vi "IRISS V2 Phaco v1.vi"() -> ()   [LabVIEW 2016]
uses:
  <vilib>/Analysis/Matrix/Datatypes/RealMatrix.ctl
  <vilib>/Math Plots/3D Math Plots/3D Scatter/3D Scatter XCtrl/3D Scatter.xctl
  Subsystems/Global Variables.vi
  <vilib>/Utility/file.llb/Read Delimited Spreadsheet (DBL).vi
  <vilib>/FPGAPlugInAG/PXI-7833R/niLvFpga_Open_PXI-7833R.vi
  <vilib>/Utility/error.llb/Error Cluster From Error Code.vi
  <vilib>/rvi/errors/niLvFpgaAdjustHostInterfaceError.vi
  <vilib>/Math Plots/3D Math Plots/3D Scatter/3D Scatter Datatype/Public/Plot Helper (Vector).vi
  Library/mjglib/var_OCTzHomeDir.vi
  <vilib>/FPGAPlugInAG/PXI-7833R/niLvFpga_Reset_PXI-7833R.vi
  <vilib>/FPGAPlugInAG/PXI-7833R/niLvFpga_Close_PXI-7833R.vi
  <vilib>/rvi/interface/nirviOpenFPGA/nirviOpenFPGA.xnode
  FPGA Bitfiles/PhantomControlPI_FPGATarget_QuadCtr2_E2412E44.lvbitx
  IRISS_FPGA_IO.vi
  <vilib>/rvi/interface/nirviReadWriteControl/nirviReadWriteControl.xnode
  <vilib>/Math Plots/3D Math Plots/3D Plot/3D Plot Datatype/3D Plot Datatype.lvclass
  <vilib>/rvi/interface/nirviMethod/nirviMethod.xnode
  <vilib>/rvi/interface/nirviCloseFPGA/nirviCloseFPGA.xnode
  <vilib>/Analysis/Matrix/NI_Matrix.lvlib
  Functions/EyeRobotDLL.dll
  Library/KevinLibraryAll/labview2011/kevLib2011.lvlib
  <vilib>/Math Plots/3D Math Plots/3D Scatter/3D Scatter Datatype/3D Scatter Datatype.lvclass
  NiFpgaLv.dll
panel:
  out "Trajectory Cluster":T1
  in  "OCT Z PID Gains":cluster{"Kp":dbl, "Kd":dbl, "Ki":dbl}={"Kp"=0.0003, "Kd"=0.0001, "Ki"=0.01}
  out "deltaRoll":sgl
  out "deltaXYZ":sgl[](array[numeric])
  out "Online Eye Model":T2
  in  "To Regulation":bool
  out "Eye Model Cluster":T4={"X Grid"=[], "Y Grid"=[], "Za_true Surf"=[], "Iris Center"=[], "Zp_true Surf"=[], "Pinv"=[[1.0, 0.0], [0.0, 1.0]], "za_true"=5.0, "za_work"=1.0, "zp_work"=-1.0, "zp_true"=-5.0}
  out "Update Mdl & Traj":bool=TRUE
  in  "Initialize":bool caption="To M/S"
  in  "IRISS GUI":T5(tab)
  in  "U/S Power [%]":sgl min=0 max=100 step=10
  in  "Vac Cmd [mmHg]":sgl min=0 max=600 step=50
  in  "Red Round Box":u32(colorbox)=16711690
  in  "Blue Round Box":u32(colorbox)=16860
  in  "Black Round Box":u32(colorbox)
  out "Vacuum Force [mmHg]  2":i32 caption="[mmHg]"
  in  "IV Height [mmHg]":dbl=30.0 min=0.0 max=90.0 step=10.0
  in  "Irrigation":bool
  in  "Reroute Hold [sec]":dbl=10.0 caption="Hold [sec]"
  out "Next Speed":dbl=0.8 format="%#.2gx"
  out "Current Speed":dbl=0.2 format="%#_2gx"
  out "Next Depth":dbl=40.0 format="%#_g%%"
  out "Current Depth":dbl=20.0 format="%#_6g%%"
  in  "Depth Offset":dbl min=-30.0 max=70.0 step=5.0 format="%#_g%%"
  in  "Refractive Index":dbl=1.35
  in  "PO No-Fly":dbl=5.0 step=0.1 format="%#.2g"
  out "PO Cruising":dbl=5.0 format="%#.2g"
  in  "Iris Center":dbl=5.0 step=0.1 format="%#.2g"
  in  "AN Cruising":dbl=5.0 step=0.1 format="%#.2g"
  in  "AN No-Fly":dbl=5.0 step=0.1 format="%#.2g"
  in  "Iris XY Scaling":dbl[](array[numeric])=[1.0, 1.0] caption="Iris Scaling" min=0.5 max=2.0 step=0.05
  in  "Iris XY Center":dbl[](array[numeric])=[0.0, 5.0] caption="Iris Center" min=-5.0 max=5.0 step=0.25
  out "Asgn Pt Out of Bound":bool caption="Assign Pt OOB"
  out "Emergency alarm":bool
  out "Remote sender engaged":bool
  out "State changing":bool
  out "Current Run No.":u8
  out "No. of Runs":i32=5
  out "Tip out Posit":dbl[](array[numeric]) caption="Position [mm]" format="%#.3f"
  out "Tip cmd Posit":dbl[](array[numeric]) caption="Command [mm]" format="%#.3f"
  out "State Flag Array":bool[](array[boolean])
  in  "Speed Override":u16=3
  out "Timer":i32 format="%<%M:%S>t"
  in  "Assign Point [mm]":dbl[](array[numeric])=[0.0, -7.0, -6.0]
  in  "Go to Assign Pt":bool
  out "Irrigation Engaged?":bool caption="Irrigation Engaged"
  out "Robot XYZ":refnum<class "3D Plot Datatype.lvclass">[](xcontrol)
  in  "Offset":dbl[](array[numeric])
  in  "Radial Scale":dbl=0.5
  in  "Pattern":T6(ring)=enum."Centered"
  in  "Stop-and-Go":bool
  in  "SCAN_NO":string
  in  "Gen Traj":bool
  out "Trajectory OOB":bool
  out "Current System State":T7(ring)
  in  "Current Surgical Stage":T8(ring)
  in  "Tracking Mode":u16(ring) items=["Joint Mode", "XYZ Mode"]
  in  "Stage Z [mm]":dbl=100.0 min=-120.0 max=120.0 step=0.5
  in  "Stage Y [mm]":dbl=70.0 min=-120.0 max=100.0 step=0.5
  in  "Gripper":dbl
  in  "OCT Cmd Z [mm]":dbl min=-25.0 max=14.0 step=0.5
  out "Joint Out":dbl[](array[numeric])
  out "Robot Status Array":bool[](array[boolean])
  in  "L1 [deg]":dbl=-40.0
  in  "L2 [deg]":dbl=15.0
  in  "L3 [mm]":dbl=-5.0 step=0.1
  out "Status 2":bool[](array[boolean])
  in  "L4 [deg]":dbl=-10.0 step=0.1
  in  "Home":bool
  out "OCT Z out [mm]":dbl caption="OCT Out Z [mm]" format="%#.4f"
  in  "Tool Type":i32=6
  in  "Tool Offset [mm]":dbl=-50.68
  out "Grasp out":dbl format="%#.4g"
  in  "OCTz Home Dir":bool
  in  "Remote Control Source":u16(ring) caption="Remote Source" items=["None", "Surgical Console", "Joystick", "Rigid Joystick", "Zeiss PC", "MJG C++ Teleoperation", "A-Scan", ""]
  in  "Reset Joystick":bool caption="Encoder Reset"
  out "Send Count":u64
  out "Receive Count":u64
  out "Arm ID Ind":i32
  out "Status":bool
  in  "Stage X [mm]":dbl=30.0 min=-120.0 max=120.0 step=0.5
  out "XYZ Stage out":dbl[](array[numeric])
  out "XYZ Stage cmd":dbl[](array[numeric])
  out "DH Params":cluster{"d_DH":dbl[][], "ty":dbl[][]}
  in  "Use Online Scan":bool
  in  "Process VSCAN":bool
  in  "Restart":bool
  out "Generation Error":errorcluster
  out "Model Created":bool
  in  "Eye No":i16=1 min=1 step=1
  in  "Reroute Transit Vacf":dbl=100.0
  in  "Z Rot Axis":dbl=1.0
  in  "Z Dist Thld":dbl[](array[numeric])=[3.0, 5.0] caption="Z Distance Threshould"
  in  "Vac Extremum":dbl[](array[numeric])=[68.0, 68.0] caption="Vacuum Extremum"
  in  "Max Limit [mmHg]":dbl=600.0 min=0.0 max=600.0 step=100.0
  out "Value [mmHg]":i8
  in  "Save Data":bool
  out "File Exists":bool
  out "File Path":path
  out "Elaspsed Time [s]":sgl
  in  "Data No":i16=1 min=1 step=1
  in  "Total Time":i16=90 min=1 step=1
  in  "Min PC Gap":dbl=0.1 caption="Min PC Gap [mm]" min=0.0 max=10.0 step=0.1 format="%#.3g"
  in  "Min AC Gap":dbl=0.1 caption="Min AC Gap [mm]" min=0.0 max=10.0 step=0.1 format="%#.3g"
  out "Scaling":dbl[](array[numeric])=[1.0, 1.0, 1.0] caption="S" min=0.5 max=1.5 step=0.05 format="%#_3g"
  in  "Joint Limits":dbl[][](array[numeric])=[[-68.0, -4.0], [-26.0, 52.0], [-40.0, 23.0], [-180.0, 180.0]] format="%#.3g"
  out "First Trk Pt":dbl[](array[numeric]) format="%#.3g"
  out "Error(s) Out on Program End":errorcluster
  out "L4 Waveform Graph":dbl[](graph)
  out "L3 Waveform Graph":dbl[](graph)
  out "L2 Waveform Graph":dbl[](graph)
  out "L1 Waveform Graph":dbl[](graph)
  in  "Aiming Pt":dbl[](array[numeric])=[-40.0, 11.0, 2.0, 0.0] format="%#.3g"
  in  "Engage Pt":dbl[](array[numeric])=[-40.0, 11.0, 2.0, 0.0] format="%#.3g"
  in  "Rotation":dbl[](array[numeric])=[0.0, 0.0, 0.0] caption="R [deg]" min=-15.0 max=15.0 step=0.5 format="%#_3g"
  out "Translation":dbl[](array[numeric]) caption="T [mm]" min=-3.0 max=3.0 step=0.1 format="%#_3g"
  in  "Inc Ctrl":dbl[](array[numeric])=[0.1, 0.05, 0.05] caption="Increment Control"
  in  "Depth Ctrl Array\n(% Thickness)":dbl[](array[numeric])=[40.0, 60.0, 80.0] min=10.0 max=90.0 step=5.0 format="%#_g%%"
  in  "Load Traj":bool caption="To M/S"
  in  "MS/Auto":bool
  in  "Retract":bool caption="To M/S"
  in  "Stop Accurus":bool caption="To M/S"
  in  "L3 Go Home":bool caption="To M/S"
  in  "Track":bool caption="To M/S"
  in  "Insert":bool caption="To M/S"
  in  "Program Stop":bool
  # "M/S\n \nAuto"
  # "Tool Tip Location"
  # "Tracking Planning"
  # "RCM"
  # "X\nY\nZ"
  # "X\nY\nZ"
  # "Tool"
  # "Trajectory"
  # "System Progress"
  # "Assign Point Rerouting"
  # "Trajectory Generation"
  # "X\nY\nZ"
  # "X Offset"
  # "Y Offset"
  # "Homing finished"
  # "Z Offset"
  # "M/S initialization finished"
  # "Tool Cruising Boundaries"
  # "XY-plane"
  # "Trajecoty loading finished"
  # "Aiming finished"
  # "Tool engaged"
  # "Z-axis"
  # "Phaco Machine"
  # "Tracking initialization finished"
  # "In Tracking"
  # "Rerouting finished"
  # "X\nY"
  # "X\nY"
  # "In regulation"
  # "Robot Control"
  # "Homing"
  # "Joint Definition"
  # "Arm"
  # "Tool"
  # "Stage"
  # "Robot Status"
  # "Joint M/S Cmd"
  # "HARDWARE_NOT_PRESENT"
  # "HARDWARE_NOT_FOUND_ALL_DRIVES"
  # "HARDWARE_SENSOR_FAULT"
  # "NOT_RUNNING"
  # "COMMUNICATION_ERROR"
  # "KINEMATICS_NO_SOLUTION"
  # "OCT Control"
  # "KINEMATICS_INSERTION_LENGTH_TOO_SMALL"
  # "COMMAND_BEYOND_JOINT_RANGE"
  # "COMMAND_TOO_LARGE"
  # "Eye Model Creation"
  # "Irrigation and Aspiration"
  # "IOP Control"
  # "Data Saving"
  # "Irrigation"
  # "Aspiration"
  # "ACh"
  # "Vitreous"
  # "Rotation & Vacuum Force Scheduling"
  # "Joint Motion & Control"
  # "Space Deform Parameters"
  # "Depth Ctrl"
  # "S"
  # "R"
  # "[deg]"
  # "T"
  # "[mm]"
  # "First Track Point"
  # "AC & PC Gap"
  # "X1"
  # "[mm]"
  # "Y"
  # "[mm]"
  # "Z"
  # "[mm]"
  # "L4"
  # "[deg]"
  # "Joint Limits"
  # "Error Message"
  # "Incision"
  # "Min."
  # "Max."
  # "L1"
  # "[deg]"
  # "L1"
  # "L2"
  # "L2"
  # "[deg]"
  # "L3"
  # "[mm]"
  # "L3"
  # "L4"
  # "[deg]"
  # "L4"
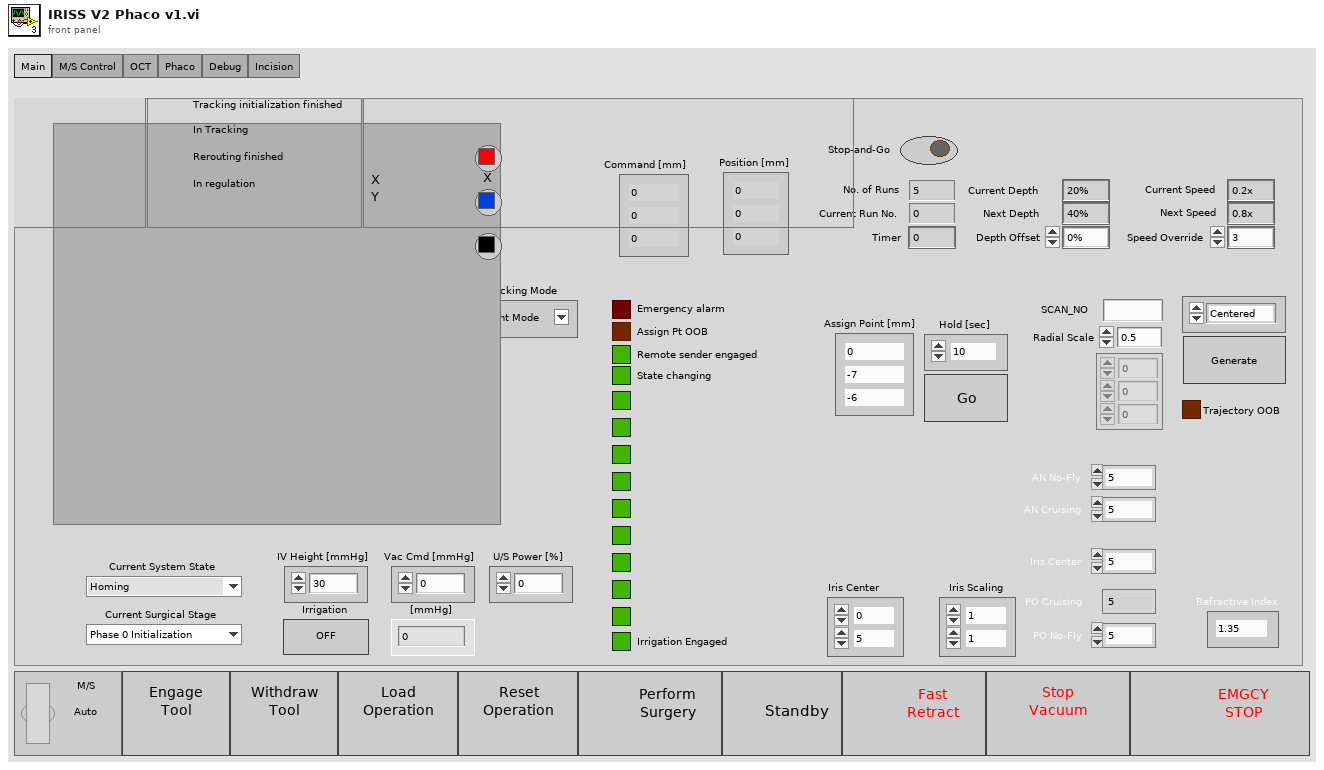
[diagram p1: front panel]
types:
  T1 = cluster{"Traj Px Array":dbl[], "Traj Py Array":dbl[], "Traj Pz Array":dbl[], "Speed Array":dbl[], "Depth Array":dbl[], "Traj Joint1 Array":dbl[], "Traj Joint2 Array":dbl[], "Traj Joint3 Array":dbl[], "Traj Joint4 Array":dbl[], "Traj Joint5 Array":dbl[]}
  T2 = cluster{"za_true":dbl, "za_work":dbl, "zi":dbl, "zp_work":dbl, "zp_true":dbl, "Iris XY Center":dbl[], "Iris XY Scaling":dbl[]}
  T3 = typedef "NI_Matrix.lvlib/RealMatrix.ctl" = dbl[][]
  T4 = cluster{"X Grid":dbl[], "Y Grid":dbl[], "Za_true Surf":dbl[][], "Iris Center":dbl[], "Zp_true Surf":dbl[][], "Pinv":T3, "za_true":dbl, "za_work":dbl, "zp_work":dbl, "zp_true":dbl}
  T5 = enum32{"Main", "M/S Control", "OCT", "Phaco", "Debug", "Incision"}
  T6 = enum16{"Entry Site", "Centered", "Insertion", "Extraction", "Reverse Entry Site", "Reverse Centered"}
  T7 = enum16{"Homing", "M/S Initialization", "M/S Operation", "Aiming", "Engaging", "Trajectory Loading", "Tracking Initialization", "Tracking", "Rerouting", "Regulation"}
  T8 = enum16{"Phase 0 Initialization", "Phase 1 Phaco", "Phase 2 Lens Removal", "Phase 3 IOL Injection"}
  T9 = enum8{"Enabled", "Disabled", "Disabled and Grayed Out"}
  T10 = cluster{"za_true_0":dbl, "za_work_0":dbl, "zp_work_0":dbl, "zp_true_0":dbl, "IrisCenter_0":dbl[]}
  T11 = cluster{"X Grid":dbl[], "Y Grid":dbl[], "Za_true Surf":dbl[][], "Iris Center":dbl[], "Zp_true Surf":dbl[][], "Real Matrix":T3, "za_true":dbl, "za_work":dbl, "zp_work":dbl, "zp_true":dbl}
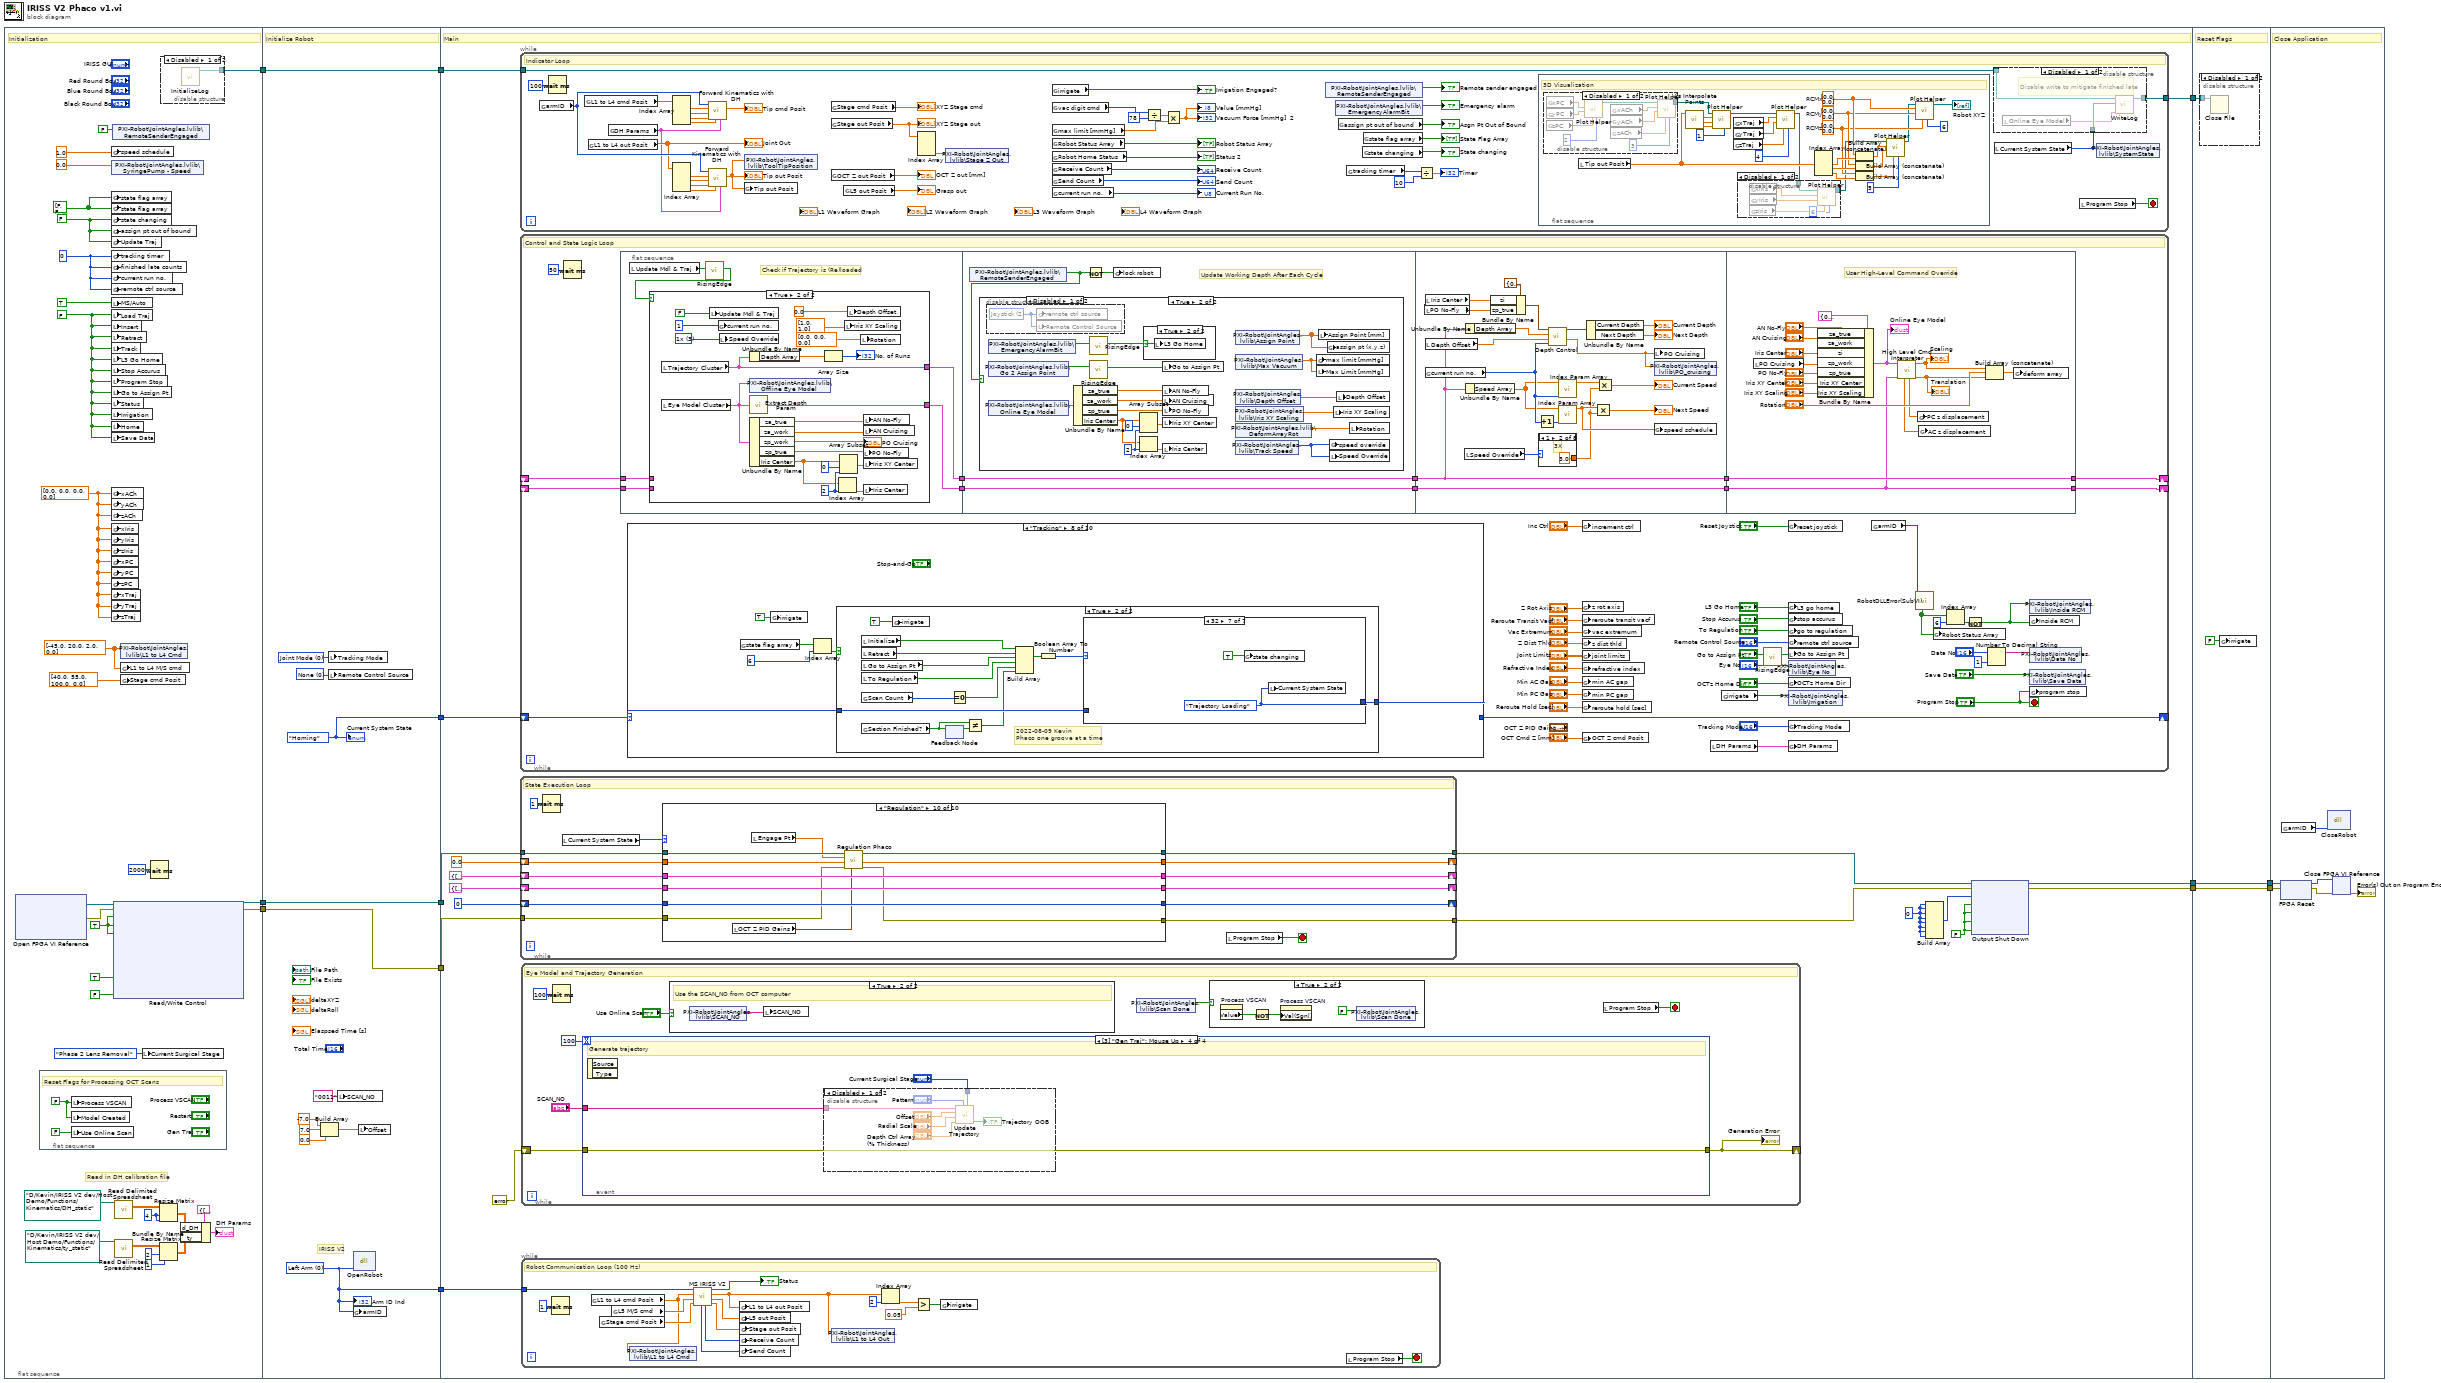
[diagram p0: block diagram]
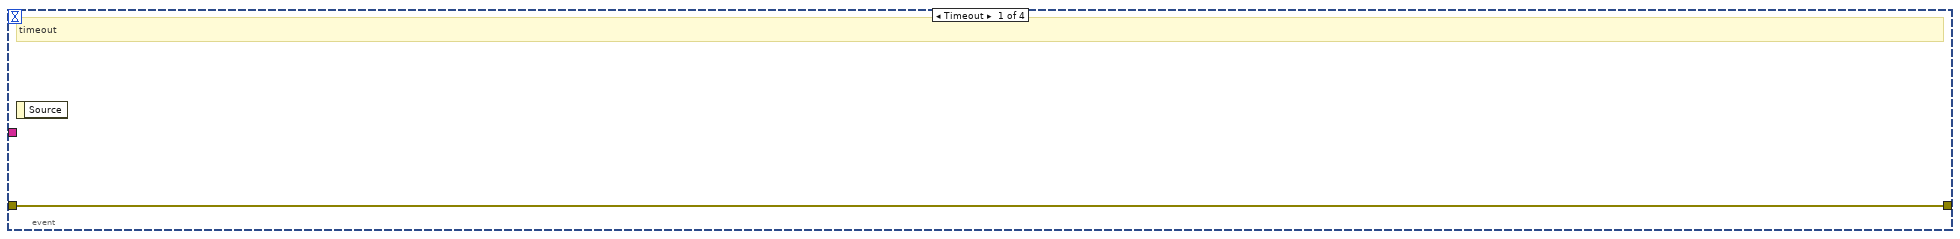
[diagram p5: hidden frame]
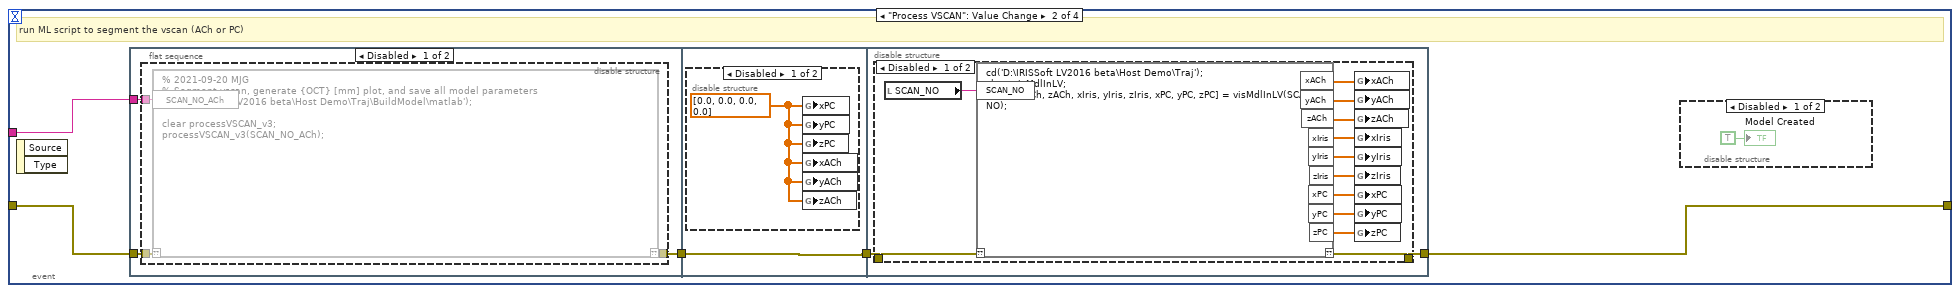
[diagram p6: hidden frame]
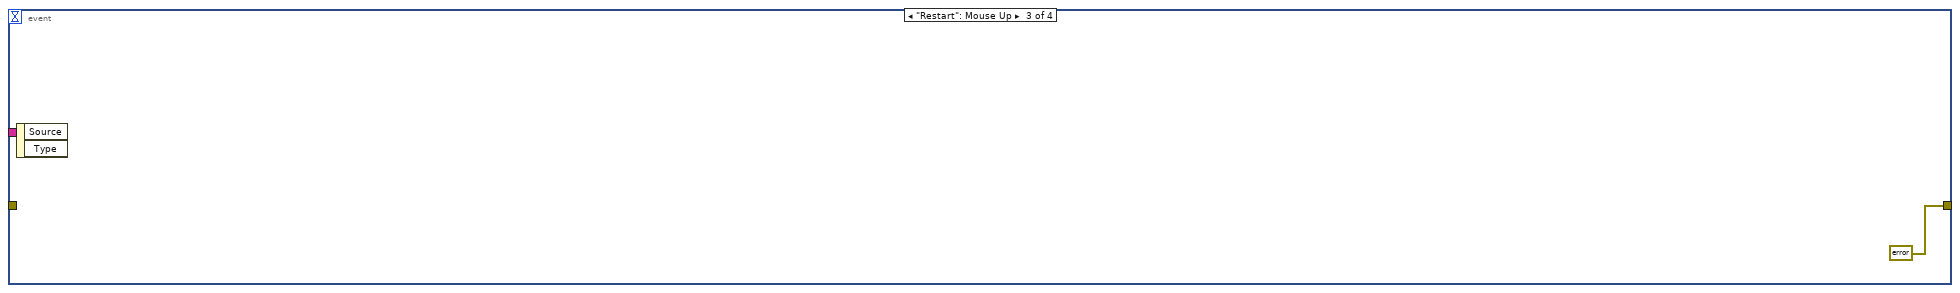
[diagram p11: hidden frame]
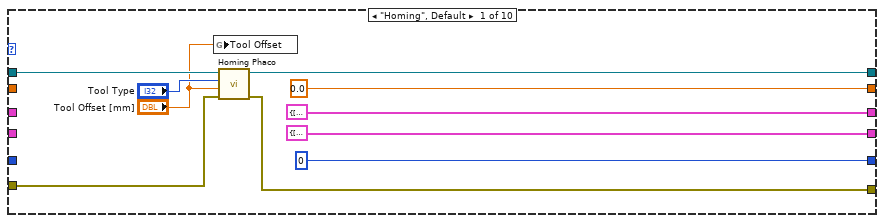
[diagram p13: hidden frame]
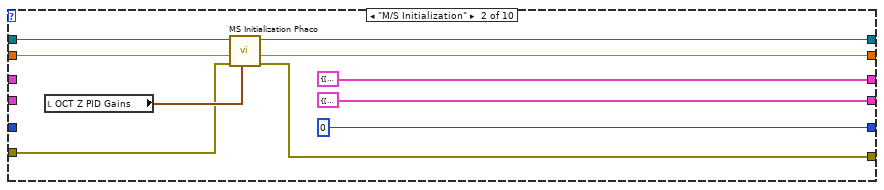
[diagram p14: hidden frame]
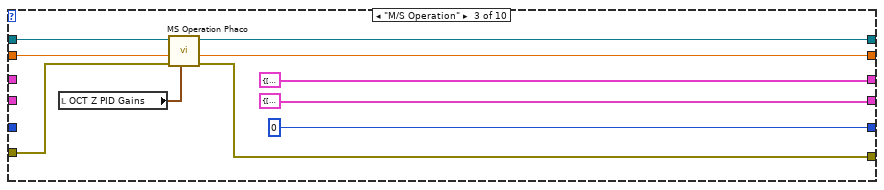
[diagram p15: hidden frame]
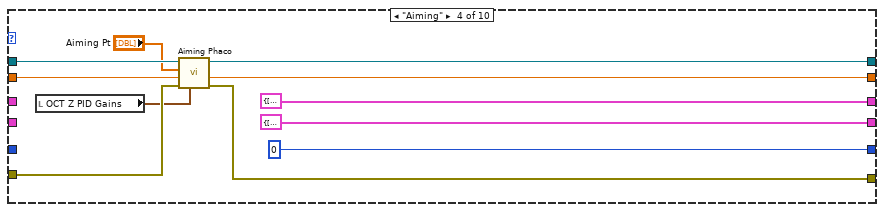
[diagram p16: hidden frame]
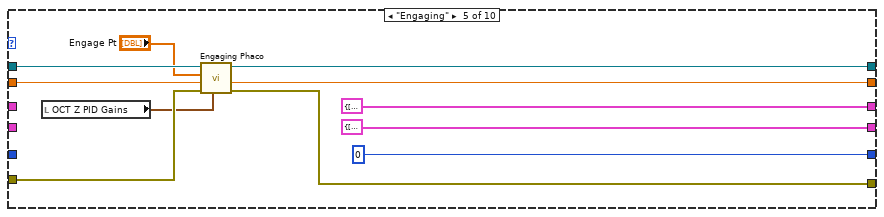
[diagram p17: hidden frame]
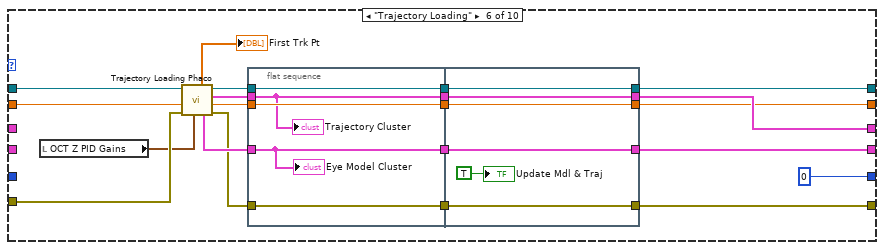
[diagram p18: hidden frame]
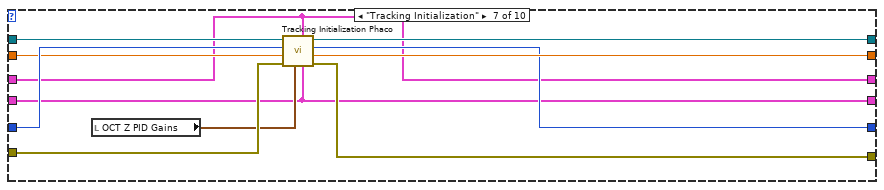
[diagram p19: hidden frame]
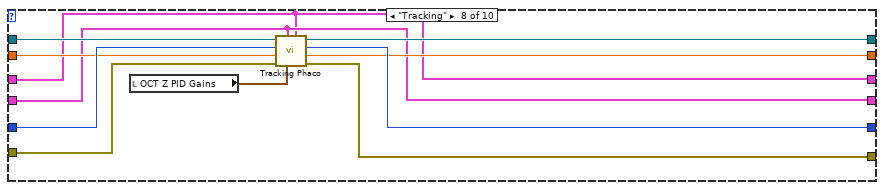
[diagram p20: hidden frame]
diagram:
  n1 = flat-sequence {
    tunnel: [w44] -> w5
    tunnel: [w36] -> w3
    tunnel: [w35] -> w2
    tunnel: [w58] -> w8
    tunnel: [w59] -> w7
    tunnel: [w57] -> w6
    tunnel: w5 -> [w60]
    tunnel: [w60] -> w4
    tunnel: w3 -> [w59]
    tunnel: w2 -> [w58]
    tunnel: [w50] -> w1
    tunnel: w8 -> [w75]
    tunnel: w7 -> [w72]
    tunnel: w6 -> [w78]
    tunnel: [w73] -> w13
    tunnel: [w74] -> w12
    tunnel: w4 -> [w77]
    tunnel: [w76] -> w11
    tunnel: w1 -> [w63]
    tunnel: w13 -> [w818]
    tunnel: w12 -> [w819]
    tunnel: w11 -> [w820]
    tunnel: [w819] -> w10
    tunnel: [w818] -> w9
    tunnel: w10 -> [w827]
    tunnel: w9 -> [w826]
    frame #0 {
      w22 = 4 ("number of rows")
      w37 = TRUE ("Conn0/DIO13 Button 2")
      w33 = dbl[] [0.0, 0.0, 0.0, 0.0] ("First Trk Pt 2")
      w28 = dbl[] [-45.0, 20.0, 2.0, 0.0] ("First Trk Pt 2")
      w32 = 0 ("finished late counts")
      w43 = bool[] [FALSE, FALSE, FALSE, FALSE, FALSE, FALSE, FALSE, FALSE, FALSE] ("state flag array")
      w41 = FALSE ("state changing")
      w34 = FALSE ("program stop")
      # "Read in DH calibration file"
      # "Initialization"
      n2 = xnode "Open FPGA VI Reference"() -> ("FPGA VI Reference Out"=w31:refnum<k20>, "error out"=w30:errorcluster)  [unwired: 2 in]
      n3 = flat-sequence {
        frame #0 {
          w46 = FALSE ("ACh Processed")
          # "Reset Flags for Processing OCT Scans"
          n4 = local write "Process VSCAN"(w46) -> ()
          n5 = local write "Model Created"(w46) -> ()
          n6 = local write "Use Online Scan"(FALSE ("Use Online Scan")) -> ()
        }
      }
      n7 = global write "Global Variables.vi" "speed schedule"(1.0 ("speed schedule")) -> ()
      n8 = shared-variable "PXI-Robot\\JointAngles.lvlib\\SyringePump - Speed"(0.0 ("SyringePump - Speed")) -> ()  [unwired: 1 in, 1 out]
      n9 = global write "Global Variables.vi" "state flag array"(w43) -> ()
      n10 = global write "Global Variables.vi" "state flag array"(w43) -> ()
      n11 = global write "Global Variables.vi" "state changing"(w41) -> ()
      n12 = global write "Global Variables.vi" "assign pt out of bound"(w41) -> ()
      n13 = global write "Global Variables.vi" "Update Traj"(w41) -> ()
      n14 = global write "Global Variables.vi" "tracking timer"(w32) -> ()
      n15 = global write "Global Variables.vi" "finished late counts"(w32) -> ()
      n16 = global write "Global Variables.vi" "current run no."(w32) -> ()
      n17 = global write "Global Variables.vi" "remote ctrl source"(w32) -> ()
      n18 = local write "MS/Auto"(TRUE ("MS/Auto")) -> ()
      n19 = local write "Load Traj"(w34) -> ()
      n20 = local write "Insert"(w34) -> ()
      n21 = local write "Retract"(w34) -> ()
      n22 = local write "Track"(w34) -> ()
      n23 = local write "L3 Go Home"(w34) -> ()
      n24 = local write "Stop Accurus"(w34) -> ()
      n25 = local write "Program Stop"(w34) -> ()
      n26 = local write "Go to Assign Pt"(w34) -> ()
      n27 = local write "Status"(w34) -> ()
      n28 = local write "Irrigation"(w34) -> ()
      n29 = local write "Home"(w34) -> ()
      n30 = local write "Save Data"(w34) -> ()
      n31 = global write "Global Variables.vi" "xACh"(w33) -> ()
      n32 = global write "Global Variables.vi" "yACh"(w33) -> ()
      n33 = global write "Global Variables.vi" "zACh"(w33) -> ()
      n34 = global write "Global Variables.vi" "xIris"(w33) -> ()
      n35 = global write "Global Variables.vi" "yIris"(w33) -> ()
      n36 = global write "Global Variables.vi" "zIris"(w33) -> ()
      n37 = global write "Global Variables.vi" "xPC"(w33) -> ()
      n38 = global write "Global Variables.vi" "yPC"(w33) -> ()
      n39 = global write "Global Variables.vi" "zPC"(w33) -> ()
      n40 = global write "Global Variables.vi" "xTraj"(w33) -> ()
      n41 = global write "Global Variables.vi" "yTraj"(w33) -> ()
      n42 = global write "Global Variables.vi" "zTraj"(w33) -> ()
      n43 = shared-variable "PXI-Robot\\JointAngles.lvlib\\RemoteSenderEngaged"(FALSE ("RemoteSenderEngaged")) -> ()  [unwired: 1 in, 1 out]
      n44 = xnode "Read/Write Control"("FPGA VI Reference In"=w31, "error in"=w30, "Conn0/DIO12 Button 1"=w37, "Conn0/DIO13 Button 2"=w37, "Conn0/DIO15 Button 4"=w37, "Reset 14"=TRUE, "Hydration On/Off (Connector2/DIO28)"=FALSE) -> ("FPGA VI Reference Out"=w36:refnum<k20>, "error out"=w35:errorcluster)  [unwired: 3 in, 2 out]
      n45 = call-poly <vilib>:"Read Delimited Spreadsheet.vi"("file path (dialog if empty)"=path "D:/Kevin/IRISS V2 dev/Host Demo/Functions/Kinematics/DH_static" ("file path (use dialog)")) -> ("all rows"=w23:dbl[][])  [unwired: 9 in, 5 out]
      n46 = call-poly <vilib>:"Read Delimited Spreadsheet.vi"("file path (dialog if empty)"=path "D:/Kevin/IRISS V2 dev/Host Demo/Functions/Kinematics/ty_static" ("file path (use dialog)")) -> ("all rows"=w21:dbl[][])  [unwired: 9 in, 5 out]
      n47 = shared-variable "PXI-Robot\\JointAngles.lvlib\\L1 to L4 Cmd"(w28) -> ()  [unwired: 1 in, 1 out]
      n48 = global write "Global Variables.vi" "L1 to L4 M/S cmd"(w28) -> ()
      n49 = global write "Global Variables.vi" "Stage cmd Posit"(dbl[] [40.0, 55.0, 100.0, 0.0] ("First Trk Pt 2")) -> ()
      n50 = local write "Current Surgical Stage"(T8."Phase 2 Lens Removal" ("Current Surgical Stage")) -> ()
      n51 = Wait (ms)(milliseconds to wait=u32 2000) -> ()  [unwired: 1 out]
      n52 = Resize Matrix(1:w22, 2:w22, 4:w23) -> (0:w17:dbl[][])
      n53 = Resize Matrix(1:1 ("number of columns"), 2:2 ("number of rows"), 4:w21) -> (0:w16:dbl[][])
      n54 = disable-structure shown="Disabled" {
        disable-tunnel: [w48 _] -> w44
        frame Disabled {
          n55 = call "InitializeLog.vi"() -> ("Byte Stream File out"=w48:refnum<file>)  [unwired: 11 in]
        }
        frame Enabled {
        }
      }
      n56 = Bundle By Name(cluster=cluster{"d_DH":dbl[][], "ty":dbl[][]} {"d_DH"=[[0.0, -0.04858099004841317, 1.1971672750675049, 0.0], [0.0, -1.576475511297109, 0.0, 0.0], [-0.3552491783526254, 0.0, -1.1064589410656984, 0.2058446720735121], [-1.0573457532495087, 1.0278049025155533, 0.011917110633363169, -0.004023577880993236]], "ty"=[[0.04320445582455471], [0.011728642746432275]]} ("input cluster"), "d_DH"=w17, "ty"=w16) -> (→"DH Params":cluster{"d_DH":dbl[][], "ty":dbl[][]})
    }
    frame #1 {
      w49 = u16 0 items=["Joint Mode", "XYZ Mode"] ("Tracking Mode")
      w56 = u16 0 items=["None", "Surgical Console", "Joystick", "MJG Teleoperation", "MJG C++ Teleoperation"] ("Remote Control Source 2")
      w57 = T7."Homing" ("Current State")
      w50 = 0 items=["Left Arm", "Right Arm"] ("Left or Right Arm")
      # "IRISS V2"
      # "Initialize Robot"
      n57 = Build Array(-7.0 ("element"), 7.0 ("element"), 0.0 ("element")) -> (w55:dbl[])
      n58 = local write "Tracking Mode"(w49) -> ()
      n59 = local write "Remote Control Source"(w56) -> ()
      n60 = local write "SCAN_NO"("0011" ("SCAN_NO")) -> ()
      n61 = dll-call lib="D:/Kevin/IRISS V2 dev/Host Demo/Functions/EyeRobotDLL.dll" fn="OpenRobot" label="Open"("id"=w50) -> ()  [unwired: 5 in, 2 out]
      n62 = global write "Global Variables.vi" "armID"(w50) -> ()
      n63 = local write "Offset"(w55) -> ()
      "Arm ID Ind" <- w50
      "Current System State" <- w57
    }
    frame #2 {
      w66 = FALSE
      w64 = i16 0 ("element")
      # "Main"
      n64 = while {
        shift-right: [w415] -> _
        shift-left: w78 -> [w416]
        shift-right: [w412] -> _
        shift-left: _ -> [w410]
        shift-right: [w411] -> _
        shift-left: _ -> [w409]
        stop <- "Program Stop" stop-if-true
        # "Control and State Logic Loop"
        n65 = Wait (ms)(milliseconds to wait=u32 50) -> ()  [unwired: 1 out]
        n66 = flat-sequence {
          tunnel: [w429] -> w401
          tunnel: [w428] -> w400
          tunnel: w410 -> [w427]
          tunnel: w409 -> [w426]
          tunnel: w401 -> [w457]
          tunnel: w400 -> [w456]
          tunnel: [w457] -> w399
          tunnel: [w456] -> w398
          tunnel: w399 -> [w485]
          tunnel: [w485] -> w397
          tunnel: w398 -> [w502]
          tunnel: [w502] -> w396
          tunnel: w397 -> [w525]
          tunnel: w396 -> [w515]
          tunnel: [w515] -> w411
          tunnel: [w525] -> w412
          frame #0 {
            # "Check if Trajectory is (Re)loaded"
            n67 = local read "Update Mdl & Traj"() -> (w431:bool)
            n68 = call "RisingEdge.vi"("Signal In"=w431) -> ("Rising Edge"=w430:bool)  [unwired: 10 in]
            n69 = case shown="True" w430 {
              tunnel: [w432 w453] -> w428
              tunnel: [w433 w442] -> w429
              tunnel: w427 -> [w433 _]
              tunnel: w426 -> [w432 _]
              frame False {
                # "Use Nominal Model & Trajectory"
              }
              frame True {
                w435 = u16 3 items=["4x", "3x", "2x", "1x", "0.5x", "0.2x", "0.1x", "PAUSE"] ("Speed Override")
                w447 = 2 ("index")
                # "Update Trajectory and Model after \"Trajectory Loading\""
                n70 = local read "Trajectory Cluster"() -> (w442:T1)
                n71 = local read "Eye Model Cluster"() -> (w440:T4)
                n72 = local write "Update Mdl & Traj"(FALSE ("Update Model")) -> ()
                n73 = global write "Global Variables.vi" "current run no."(u8 1 ("current run no.")) -> ()
                n74 = local write "Speed Override"(w435) -> ()
                n75 = Unbundle By Name(w442) -> ("Depth Array"=w444:dbl[])
                n76 = shared-variable "PXI-Robot\\JointAngles.lvlib\\Offline Eye Model"(w440) -> ()  [unwired: 1 in, 1 out]
                n77 = call "Extract Depth Param.vi"("Eye Model Cluster"=w440) -> ("Nominal Model param"=w453:T10)
                n78 = Unbundle By Name(w440) -> ("za_true"=w452:dbl, "za_work"=w451:dbl, "zp_work"=→"PO Cruising":dbl, "zp_true"=w449:dbl, "Iris Center"=w446:dbl[])
                n79 = Array Size(array=w444) -> (size(s)=→"No. of Runs":i32)
                n80 = Index Array(array=w446, index=w447) -> (element=w450:dbl)
                n81 = Array Subset(array=w446, index=0, length=w447) -> (w445:dbl[])
                n82 = local write "Iris XY Scaling"(dbl[] [1.0, 1.0]) -> ()
                n83 = local write "Depth Offset"(0.0 ("Depth Offset")) -> ()
                n84 = local write "Rotation"(dbl[] [0.0, 0.0, 0.0]) -> ()
                n85 = local write "PO No-Fly"(w449) -> ()
                n86 = local write "AN No-Fly"(w452) -> ()
                n87 = local write "AN Cruising"(w451) -> ()
                n88 = local write "Iris XY Center"(w445) -> ()
                n89 = local write "Iris Center"(w450) -> ()
              }
            }
          }
          frame #1 {
            # "Update Working Depth After Each Cycle"
            n90 = shared-variable "PXI-Robot\\JointAngles.lvlib\\RemoteSenderEngaged"() -> (w454:bool)  [unwired: 1 in, 1 out]
            n91 = case shown="True" w454 {
              frame False {
                n92 = global write "Global Variables.vi" "assign pt (x,y,z)"("Assign Point [mm]") -> ()
                n93 = global write "Global Variables.vi" "max limit [mmHg]"("Max Limit [mmHg]") -> ()
                n94 = global write "Global Variables.vi" "speed override"("Speed Override") -> ()
              }
              frame True {
                w465 = 2 ("index")
                n95 = disable-structure shown="Disabled" {
                  frame Disabled {
                    w480 = u16 2 items=["None", "Surgical Console", "Joystick", "MJG Teleoperation", "MJG C++ Teleoperation"] ("Remote Control Source 2")
                    n96 = global write "Global Variables.vi" "remote ctrl source"(w480) -> ()
                    n97 = local write "Remote Control Source"(w480) -> ()
                  }
                  frame Enabled {
                  }
                }
                n98 = shared-variable "PXI-Robot\\JointAngles.lvlib\\EmergencyAlarmBit"() -> (w477:bool)  [unwired: 1 in, 1 out]
                n99 = shared-variable "PXI-Robot\\JointAngles.lvlib\\Go 2 Assign Point"() -> (w474:bool)  [unwired: 1 in, 1 out]
                n100 = shared-variable "PXI-Robot\\JointAngles.lvlib\\Online Eye Model"() -> (w470:T11)  [unwired: 1 in, 1 out]
                n101 = Unbundle By Name(w470) -> ("za_true"=w473:dbl, "za_work"=w472:dbl, "zp_true"=w471:dbl, "Iris Center"=w462:dbl[])
                n102 = call "RisingEdge.vi"("Signal In"=w477) -> ("Rising Edge"=w476:bool)  [unwired: 10 in]
                n103 = call "RisingEdge.vi"("Signal In"=w474) -> ("Rising Edge"=w475:bool)  [unwired: 10 in]
                n104 = Index Array(array=w462, index=w465) -> (element=w463:dbl)
                n105 = Array Subset(array=w462, index=0, length=w465) -> (w466:dbl[])
                n106 = case shown="True" w476 {
                  selector: w476 -> [_ w481]
                  frame False {
                  }
                  frame True {
                    n107 = local write "L3 Go Home"(w481) -> ()
                  }
                }
                n108 = local write "Go to Assign Pt"(w475) -> ()
                n109 = local write "AN No-Fly"(w473) -> ()
                n110 = local write "AN Cruising"(w472) -> ()
                n111 = local write "PO No-Fly"(w471) -> ()
                n112 = local write "Iris XY Center"(w466) -> ()
                n113 = local write "Iris Center"(w463) -> ()
                n114 = shared-variable "PXI-Robot\\JointAngles.lvlib\\Assign Point"() -> (w478:dbl[])  [unwired: 1 in, 1 out]
                n115 = shared-variable "PXI-Robot\\JointAngles.lvlib\\Max Vacuum"() -> (w461:dbl)  [unwired: 1 in, 1 out]
                n116 = shared-variable "PXI-Robot\\JointAngles.lvlib\\Depth Offset"() -> (w469:dbl)  [unwired: 1 in, 1 out]
                n117 = shared-variable "PXI-Robot\\JointAngles.lvlib\\Iris XY Scaling"() -> (w468:dbl[])  [unwired: 1 in, 1 out]
                n118 = shared-variable "PXI-Robot\\JointAngles.lvlib\\DeformArrayRot"() -> (w467:dbl[])  [unwired: 1 in, 1 out]
                n119 = shared-variable "PXI-Robot\\JointAngles.lvlib\\Track Speed"() -> (w479:u16)  [unwired: 1 in, 1 out]
                n120 = global write "Global Variables.vi" "max limit [mmHg]"(w461) -> ()
                n121 = local write "Max Limit [mmHg]"(w461) -> ()
                n122 = local write "Assign Point [mm]"(w478) -> ()
                n123 = global write "Global Variables.vi" "assign pt (x,y,z)"(w478) -> ()
                n124 = global write "Global Variables.vi" "speed override"(w479) -> ()
                n125 = local write "Speed Override"(w479) -> ()
                n126 = local write "Iris XY Scaling"(w468) -> ()
                n127 = local write "Depth Offset"(w469) -> ()
                n128 = local write "Rotation"(w467) -> ()
              }
            }
            n129 = Not(x=w454) -> (.not. x?=w455:bool)
            n130 = global write "Global Variables.vi" "lock robot"(w455) -> ()
          }
          frame #2 {
            n131 = local read "PO No-Fly"() -> (w496:dbl)
            n132 = local read "Iris Center"() -> (w497:dbl)
            n133 = local read "Depth Offset"() -> (w501:dbl)
            n134 = global read "Global Variables.vi" "current run no."() -> (w494:u8)
            n135 = local read "Speed Override"() -> (w491:u16)
            n136 = Unbundle By Name(w485) -> ("Speed Array"=w493:dbl[])
            n137 = Unbundle By Name(w485) -> ("Depth Array"=w492:dbl[])
            n138 = Bundle By Name(cluster=cluster{"zi":dbl, "zp_true":dbl} {"zi"=0.0, "zp_true"=-2.5} ("z Cluster"), "zi"=w497, "zp_true"=w496) -> (w483:cluster{"zi":dbl, "zp_true":dbl})
            n139 = Increment(x=w494) -> (x+1=w495:u8)
            n140 = case shown="1" w491 {
              tunnel: [4.0 ("y") 3.0 ("y") 2.0 ("y") 1.0 ("y") 0.5 ("y") 0.2 ("y") 0.1 ("y") 0.0 ("y")] -> w488
              frame 0 {
                # "4X"
              }
              frame 1 {
                # "3X"
              }
              frame 2 {
                # "2X"
              }
              frame 3, Default {
                # "1x"
              }
              frame 4 {
                # "0.5x"
              }
              frame 5 {
                # "0.2x"
              }
              frame 6 {
                # "0.1x"
              }
              frame 7 {
                # "Pause"
              }
            }
            n141 = call "Depth Control.vi"("Current Run No."=w494, "Depth Offset"=w501, "Depth Array"=w492, "z Cluster"=w483) -> ("zp_work"=w482:dbl, "Schedule Depth & Speed"=w500:cluster{"Next Depth":dbl, "Current Depth":dbl})  [unwired: 6 in]
            n142 = call "Index Param Array.vi"("Index"=w494, "Array Input"=w493) -> ("Index Output"=w489:dbl)  [unwired: 9 in]
            n143 = call "Index Param Array.vi"("Index"=w495, "Array Input"=w493) -> ("Index Output"=w490:dbl)  [unwired: 9 in]
            n144 = Unbundle By Name(w500) -> ("Current Depth"=→"Current Depth":dbl, "Next Depth"=→"Next Depth":dbl)
            n145 = Multiply(x=w490, y=w488) -> (x*y=→"Next Speed":dbl)
            n146 = Multiply(x=w489, y=w488) -> (x*y=→"Current Speed":dbl)
            n147 = local write "PO Cruising"(w482) -> ()
            n148 = shared-variable "PXI-Robot\\JointAngles.lvlib\\PO_cruising"(w482) -> ()  [unwired: 1 in, 1 out]
            n149 = global write "Global Variables.vi" "speed schedule"(w490) -> ()
          }
          frame #3 {
            # "User High-Level Command Override"
            n150 = local read "PO Cruising"() -> (w517:dbl)
            n151 = Bundle By Name(cluster=T2 {"za_true"=0.0, "za_work"=0.0, "zi"=0.0, "zp_work"=0.0, "zp_true"=0.0, "Iris XY Center"=[0.0, 5.0], "Iris XY Scaling"=[1.0, 1.0]} ("High Level cmd"), "za_true"="AN No-Fly", "za_work"="AN Cruising", "zi"="Iris Center", "zp_work"=w517, "zp_true"="PO No-Fly", "Iris XY Center"="Iris XY Center", "Iris XY Scaling"="Iris XY Scaling") -> (w516:T2)
            "Online Eye Model" <- w516
            n152 = call "High Level Cmd Interpreter.vi"("Nominal Model param"=w515, "High Level cmd"=w516) -> ("Translation Array"=w512:dbl[], "Scaling Array"=w511:dbl[], "PC Displacement"=w513:dbl, "AC Displacement"=w514:dbl)  [unwired: 6 in]
            "Scaling" <- w511
            "Translation" <- w512
            n153 = global write "Global Variables.vi" "PC z displacement"(w513) -> ()
            n154 = global write "Global Variables.vi" "AC z displacement"(w514) -> ()
            n155 = Build Array (concatenate)(w511, "Rotation", w512) -> (w526:dbl[])
            n156 = global write "Global Variables.vi" "deform array"(w526) -> ()
          }
        }
        n157 = case shown="\"Tracking\"" w416 {
          selector: w416 -> [w530 w537 w563 w616 w636 w662 w671 w702 w739 w767]
          tunnel: [w529 w538 w562 w615 w637 w663 w672 w703 w740 w768] -> w415
          frame "Homing", Default {
            # "State Diagram"
            n158 = global read "Global Variables.vi" "state flag array"() -> (w531:bool[])
            n159 = Index Array(array=w531, index=0) -> (element=w528:bool)
            n160 = case shown="False" w528 {
              tunnel: [w533 w535] -> w529
              tunnel: w530 -> [w533 _]
              frame False {
                # "homing in process"
              }
              frame True {
                w535 = T7."M/S Initialization" ("Current State")
                # "finish homing"
                n161 = global write "Global Variables.vi" "state changing"(TRUE ("state changing")) -> ()
                n162 = global write "Global Variables.vi" "Enforce Homing"(FALSE ("Enforce Homing")) -> ()
                n163 = local write "Current System State"(w535) -> ()
              }
            }
          }
          frame "M/S Initialization" {
            n164 = global read "Global Variables.vi" "state flag array"() -> (w540:bool[])
            n165 = Index Array(array=w540, index=1) -> (element=w539:bool)
            n166 = case shown="False" w539 {
              tunnel: [w551 w553] -> w538
              tunnel: w537 -> [w551 _]
              frame False {
                n167 = global read "Global Variables.vi" "Stage cmd Posit"() -> (w545:dbl[])
                n168 = property on="MS/Auto" class="Bool (strict)"("DisabledEnum"=T9."Disabled and Grayed Out" ("Disabled")) -> ()  [unwired: 2 in, 2 out]
                n169 = Index Array(array=w545) -> (element #1=w543:dbl, element #2=w544:dbl, element #3=w542:dbl)  [unwired: 3 in]
                n170 = global read "Global Variables.vi" "L1 to L4 M/S cmd"() -> (w550:dbl[])
                n171 = local write "Stage X [mm]"(w543) -> ()
                n172 = local write "Stage Y [mm]"(w544) -> ()
                n173 = local write "Stage Z [mm]"(w542) -> ()
                n174 = Index Array(array=w550) -> (element #1=w549:dbl, element #2=w548:dbl, element #3=w547:dbl, element #4=w546:dbl)  [unwired: 4 in]
                n175 = local write "L1 [deg]"(w549) -> ()
                n176 = local write "L2 [deg]"(w548) -> ()
                n177 = local write "L3 [mm]"(w547) -> ()
                n178 = local write "L4 [deg]"(w546) -> ()
              }
              frame True {
                w553 = T7."M/S Operation" ("Current State")
                n179 = global write "Global Variables.vi" "state changing"(TRUE ("state changing")) -> ()
                n180 = property on="MS/Auto" class="Bool (strict)"("DisabledEnum"=T9."Enabled" ("Disabled")) -> ()  [unwired: 2 in, 2 out]
                n181 = local write "Current System State"(w553) -> ()
              }
            }
          }
          frame "M/S Operation" {
            n182 = local read "MS/Auto"() -> (w561:bool)
            n183 = local read "Load Traj"() -> (w559:bool)
            n184 = Not(x=w561) -> (.not. x?=w560:bool)
            n185 = Build Array(w560, w559, "Home") -> (w558:bool[])
            n186 = Boolean Array To Number(Boolean array=w558) -> (number=w557:u32)
            n187 = case shown="0, Default" w557 {
              tunnel: w563 -> [w566 _ w606 _]
              tunnel: [w566 w602 w607 w614] -> w562
              frame 0, Default {
                n188 = global read "Global Variables.vi" "remote ctrl source"() -> (w565:u16)
                n189 = global write "Global Variables.vi" "irrigate"("Irrigation") -> ()
                n190 = case shown="0, Default" w565 {
                  frame 0, Default {
                    n191 = Build Array("L1 [deg]", "L2 [deg]", "L3 [mm]", "L4 [deg]") -> (w582:dbl[])
                    n192 = Build Array("Stage X [mm]", "Stage Y [mm]", "Stage Z [mm]") -> (w587:dbl[])
                    n193 = global write "Global Variables.vi" "L1 to L4 M/S cmd"(w582) -> ()
                    n194 = global write "Global Variables.vi" "Stage cmd Posit"(w587) -> ()
                    n195 = global write "Global Variables.vi" "L5 M/S cmd"("Gripper") -> ()
                  }
                  frame 1 {
                    n196 = local read "OCT Cmd Z [mm]"() -> (w592:dbl)
                    n197 = global write "Global Variables.vi" "OCT Z cmd Posit"(w592) -> ()
                  }
                  frame 2 {
                    n198 = global read "Global Variables.vi" "Stage cmd Posit"() -> (w601:dbl[])
                    n199 = Index Array(array=w601) -> (element #1=w600:dbl, element #2=w599:dbl, element #3=w598:dbl)  [unwired: 3 in]
                    n200 = local write "Stage X [mm]"(w600) -> ()
                    n201 = local write "Stage Y [mm]"(w599) -> ()
                    n202 = local write "Stage Z [mm]"(w598) -> ()
                    n203 = global read "Global Variables.vi" "L1 to L4 cmd Posit"() -> (w593:dbl[])
                    n204 = Index Array(array=w593) -> (element #1=w596:dbl, element #2=w595:dbl, element #3=w594:dbl, element #4=w597:dbl)  [unwired: 4 in]
                    n205 = local write "L1 [deg]"(w596) -> ()
                    n206 = local write "L2 [deg]"(w595) -> ()
                    n207 = local write "L3 [mm]"(w594) -> ()
                    n208 = local write "L4 [deg]"(w597) -> ()
                  }
                  frame 3 {
                  }
                }
                n209 = disable-structure shown="Disabled" {
                  frame Disabled {
                    n210 = local read "Max Limit [mmHg]"() -> (w573:dbl)
                    n211 = In Range and Coerce(upper limit=w573, x="Vac Cmd [mmHg]", lower limit=0.0) -> (coerced(x)=w574:dbl)  [unwired: 1 out]
                    n212 = To Double Precision Float(number=w574) -> (double precision float=w575:dbl)
                    n213 = Divide(x=w575, y=w573) -> (x/y=w568:dbl)
                    n214 = Multiply(x="IV Height [mmHg]", y=1.36) -> (x*y=w579:dbl)
                    n215 = Multiply(x=w568, y=78.0) -> (x*y=w570:dbl)
                    n216 = To Long Integer(number=w579) -> (32bit integer=w580:i32)
                    n217 = To Long Integer(number="U/S Power [%]") -> (32bit integer=w576:i32)
                    n218 = To Byte Integer(number=w570) -> (8bit integer=w567:i8)
                    n219 = shared-variable "PXI-Robot\\JointAngles.lvlib\\Irrigation Height"(w580) -> ()  [unwired: 1 in, 1 out]
                    n220 = global write "Global Variables.vi" "us cmd"("U/S Power [%]") -> ()
                    n221 = shared-variable "PXI-Robot\\JointAngles.lvlib\\US Cmd"(w576) -> ()  [unwired: 1 in, 1 out]
                    n222 = shared-variable "PXI-Robot\\JointAngles.lvlib\\Vacuum Cmd"(w575) -> ()  [unwired: 1 in, 1 out]
                    n223 = global write "Global Variables.vi" "vac digit cmd"(w567) -> ()
                  }
                  frame Enabled {
                  }
                }
              }
              frame 1 {
                w602 = T7."Aiming" ("Current State")
                n224 = global write "Global Variables.vi" "state changing"(TRUE ("state changing")) -> ()
                n225 = local write "Current System State"(w602) -> ()
                n226 = property on="MS/Auto" class="Bool (strict)"("DisabledEnum"=T9."Disabled and Grayed Out" ("Disabled")) -> ()  [unwired: 2 in, 2 out]
              }
              frame 2 {
                n227 = global read "Global Variables.vi" "Inside RCM"() -> (w605:bool)
                n228 = case shown="True" w605 {
                  tunnel: [w608 w609] -> w607
                  tunnel: w606 -> [w608 _]
                  frame False {
                  }
                  frame True {
                    w609 = T7."Trajectory Loading" ("Current State")
                    w610 = FALSE ("MS/Auto")
                    n229 = global write "Global Variables.vi" "state changing"(TRUE ("state changing")) -> ()
                    n230 = local write "MS/Auto"(w610) -> ()
                    n231 = local write "Load Traj"(w610) -> ()
                    n232 = local write "Current System State"(w609) -> ()
                    n233 = property on="MS/Auto" class="Bool (strict)"("DisabledEnum"=T9."Disabled and Grayed Out" ("Disabled")) -> ()  [unwired: 2 in, 2 out]
                  }
                }
              }
              frame 4 {
                w614 = T7."Homing" ("Current State")
                w613 = TRUE ("state changing")
                n234 = global write "Global Variables.vi" "state changing"(w613) -> ()
                n235 = global write "Global Variables.vi" "Enforce Homing"(w613) -> ()
                n236 = local write "Current System State"(w614) -> ()
              }
            }
          }
          frame "Aiming" {
            n237 = global read "Global Variables.vi" "state flag array"() -> (w618:bool[])
            n238 = Index Array(array=w618, index=3) -> (element=w617:bool)
            n239 = case shown="True" w617 {
              tunnel: w616 -> [w620 w624]
              tunnel: [w620 w623] -> w615
              frame False {
              }
              frame True {
                n240 = property on="MS/Auto" class="Bool (strict)"("DisabledEnum"=T9."Enabled" ("Disabled")) -> ()  [unwired: 2 in, 2 out]
                n241 = Build Array("Insert", "MS/Auto") -> (w628:bool[])
                n242 = Boolean Array To Number(Boolean array=w628) -> (number=w625:u32)
                n243 = case shown="1" w625 {
                  tunnel: w624 -> [w629 _ _]
                  tunnel: [w629 w630 w634] -> w623
                  frame 0, Default {
                  }
                  frame 1 {
                    w630 = T7."Engaging" ("Current State")
                    n244 = global write "Global Variables.vi" "state changing"(TRUE ("state changing")) -> ()
                    n245 = local write "Insert"(FALSE ("Enter")) -> ()
                    n246 = property on="MS/Auto" class="Bool (strict)"("DisabledEnum"=T9."Disabled and Grayed Out" ("Disabled")) -> ()  [unwired: 2 in, 2 out]
                    n247 = local write "Current System State"(w630) -> ()
                  }
                  frame 2 {
                    w634 = T7."M/S Initialization" ("Current State")
                    n248 = global write "Global Variables.vi" "state changing"(TRUE ("state changing")) -> ()
                    n249 = local write "Current System State"(w634) -> ()
                  }
                }
                n250 = local read "OCT Cmd Z [mm]"() -> (w621:dbl)
                n251 = global write "Global Variables.vi" "OCT Z cmd Posit"(w621) -> ()
              }
            }
          }
          frame "Engaging" {
            n252 = global read "Global Variables.vi" "state flag array"() -> (w639:bool[])
            n253 = Index Array(array=w639, index=4) -> (element=w638:bool)
            n254 = case shown="True" w638 {
              tunnel: [w642 w649] -> w637
              tunnel: w636 -> [w643 w650]
              frame False {
                n255 = local read "Retract"() -> (w641:bool)
                n256 = case shown="False" w641 {
                  tunnel: [w644 w645] -> w642
                  tunnel: w643 -> [w644 _]
                  frame False {
                  }
                  frame True {
                    w645 = T7."Aiming" ("Current State")
                    n257 = global write "Global Variables.vi" "state changing"(TRUE ("state changing")) -> ()
                    n258 = local write "Retract"(FALSE ("Retract")) -> ()
                    n259 = local write "Current System State"(w645) -> ()
                  }
                }
              }
              frame True {
                n260 = Build Array("Load Traj", "Retract") -> (w653:bool[])
                n261 = Boolean Array To Number(Boolean array=w653) -> (number=w651:u32)
                n262 = case shown="2" w651 {
                  tunnel: w650 -> [w654 _ _]
                  tunnel: [w654 w655 w658] -> w649
                  frame 0, Default {
                  }
                  frame 1 {
                    w655 = T7."Trajectory Loading" ("Current State")
                    n263 = global write "Global Variables.vi" "state changing"(TRUE ("state changing")) -> ()
                    n264 = local write "Load Traj"(FALSE ("Load Traj")) -> ()
                    n265 = local write "Current System State"(w655) -> ()
                  }
                  frame 2 {
                    w658 = T7."Aiming" ("Current State")
                    n266 = global write "Global Variables.vi" "state changing"(TRUE ("state changing")) -> ()
                    n267 = local write "Retract"(FALSE ("Load Traj")) -> ()
                    n268 = local write "Current System State"(w658) -> ()
                  }
                }
              }
            }
          }
          frame "Trajectory Loading" {
            n269 = global read "Global Variables.vi" "state flag array"() -> (w665:bool[])
            n270 = global write "Global Variables.vi" "irrigate"(TRUE ("irrigate")) -> ()
            n271 = Index Array(array=w665, index=2) -> (element=w664:bool)
            n272 = case shown="False" w664 {
              tunnel: [w667 w668] -> w663
              tunnel: w662 -> [w667 _]
              frame False {
              }
              frame True {
                w668 = T7."Tracking Initialization" ("Current State")
                n273 = global write "Global Variables.vi" "state changing"(TRUE ("state changing")) -> ()
                n274 = local write "Current System State"(w668) -> ()
              }
            }
          }
          frame "Tracking Initialization" {
            n275 = global read "Global Variables.vi" "state flag array"() -> (w674:bool[])
            n276 = Index Array(array=w674, index=5) -> (element=w673:bool)
            n277 = case shown="True" w673 {
              tunnel: [w676 w683] -> w672
              tunnel: w671 -> [w676 w682]
              frame False {
              }
              frame True {
                n278 = local read "Load Traj"() -> (w684:bool)
                n279 = local read "Retract"() -> (w678:bool)
                n280 = local read "To Regulation"() -> (w677:bool)
                n281 = Or(x="Initialize", y=w678) -> (x .or. y?=w680:bool)
                n282 = Build Array("Track", w684, w680, w677) -> (w686:bool[])
                n283 = Boolean Array To Number(Boolean array=w686) -> (number=w685:u32)
                n284 = case shown="1" w685 {
                  tunnel: [w687 w688 w691 w694 w697] -> w683
                  tunnel: w682 -> [w687 _ _ _ _]
                  frame 0, Default {
                  }
                  frame 1 {
                    w688 = T7."Tracking" ("Current State")
                    n285 = global write "Global Variables.vi" "state changing"(TRUE ("state changing")) -> ()
                    n286 = local write "Track"(FALSE ("Track")) -> ()
                    n287 = local write "Current System State"(w688) -> ()
                  }
                  frame 2 {
                    w691 = T7."Trajectory Loading" ("Current State")
                    n288 = global write "Global Variables.vi" "state changing"(TRUE ("state changing")) -> ()
                    n289 = local write "Load Traj"(FALSE ("Load Traj")) -> ()
                    n290 = local write "Current System State"(w691) -> ()
                  }
                  frame 4 {
                    w694 = T7."Engaging" ("Current State")
                    n291 = global write "Global Variables.vi" "state changing"(TRUE ("state changing")) -> ()
                    n292 = local write "Initialize"(FALSE ("Load Traj")) -> ()
                    n293 = local write "Current System State"(w694) -> ()
                  }
                  frame 8 {
                    w697 = T7."Tracking" ("Current State")
                    w698 = FALSE  # Reset
                    n294 = global write "Global Variables.vi" "state changing"(TRUE ("state changing")) -> ()
                    n295 = local write "Track"(FALSE ("Track")) -> ()
                    n296 = local write "Current System State"(w697) -> ()
                    n297 = local write "To Regulation"(w698) -> ()
                  }
                }
              }
            }
            n298 = global write "Global Variables.vi" "irrigate"(TRUE ("irrigate")) -> ()
          }
          frame "Tracking" {
            n299 = global read "Global Variables.vi" "state flag array"() -> (w705:bool[])
            n300 = global write "Global Variables.vi" "irrigate"(TRUE ("irrigate")) -> ()
            n301 = Index Array(array=w705, index=6) -> (element=w704:bool)
            n302 = case shown="True" w704 {
              tunnel: [w707 w721] -> w703
              tunnel: w702 -> [w707 w720]
              frame False {
              }
              frame True {
                # "2022-08-09 Kevin\nPhaco one groove at a time"
                n303 = local read "Initialize"() -> (w717:bool)
                n304 = local read "Retract"() -> (w714:bool)
                n305 = local read "Go to Assign Pt"() -> (w715:bool)
                n306 = local read "To Regulation"() -> (w716:bool)
                n307 = global read "Global Variables.vi" "Scan Count"() -> (w709:u64)
                n308 = global read "Global Variables.vi" "Section Finished?"() -> (w710:bool)
                n309 = global write "Global Variables.vi" "irrigate"(TRUE ("irrigate")) -> ()
                n310 = feedback #1() -> (w712:bool)  [unwired: 1 in]
                n311 = feedback-in #1(w710) -> ()
                n312 = Equal To 0?(x=w709) -> (x = 0?=w708:bool)
                n313 = Not Equal?(x=w710, y=w712) -> (x != y?=w711:bool)
                n314 = Build Array(w717, w714, w715, w716, w708, w711) -> (w719:bool[])
                n315 = Boolean Array To Number(Boolean array=w719) -> (number=w718:u32)
                n316 = case shown="32" w718 {
                  tunnel: [w722 w723 w726 w729 w732 w735 w737] -> w721
                  tunnel: w720 -> [w722 _ _ _ _ _ _]
                  frame 0, Default {
                  }
                  frame 1 {
                    w723 = T7."Engaging" ("Current State")
                    n317 = global write "Global Variables.vi" "state changing"(TRUE ("state changing")) -> ()
                    n318 = local write "Initialize"(FALSE ("Load Traj")) -> ()
                    n319 = local write "Current System State"(w723) -> ()
                  }
                  frame 2 {
                    w726 = T7."Aiming" ("Current State")
                    n320 = global write "Global Variables.vi" "state changing"(TRUE ("state changing")) -> ()
                    n321 = local write "Retract"(FALSE ("Load Traj")) -> ()
                    n322 = local write "Current System State"(w726) -> ()
                  }
                  frame 4 {
                    w729 = T7."Rerouting" ("Current State")
                    n323 = global write "Global Variables.vi" "state changing"(TRUE ("state changing")) -> ()
                    n324 = local write "Go to Assign Pt"(FALSE ("Load Traj")) -> ()
                    n325 = local write "Current System State"(w729) -> ()
                  }
                  frame 8 {
                    w732 = T7."Regulation" ("Current State")
                    n326 = global write "Global Variables.vi" "state changing"(TRUE ("state changing")) -> ()
                    n327 = local write "Current System State"(w732) -> ()
                  }
                  frame 16 {
                    w735 = T7."Regulation" ("Current State")
                    w734 = TRUE ("state changing")
                    n328 = global write "Global Variables.vi" "state changing"(w734) -> ()
                    n329 = local write "To Regulation"(w734) -> ()
                    n330 = local write "Current System State"(w735) -> ()
                  }
                  frame 32 {
                    w737 = T7."Trajectory Loading" ("Current State")
                    n331 = global write "Global Variables.vi" "state changing"(TRUE ("state changing")) -> ()
                    n332 = local write "Current System State"(w737) -> ()
                  }
                }
              }
            }
          }
          frame "Rerouting" {
            n333 = global read "Global Variables.vi" "state flag array"() -> (w742:bool[])
            n334 = Index Array(array=w742, index=7) -> (element=w741:bool)
            n335 = case shown="True" w741 {
              tunnel: [w746 w760] -> w740
              tunnel: w739 -> [w745 _]
              frame False {
                n336 = shared-variable "PXI-Robot\\JointAngles.lvlib\\EmergencyAlarmBit"() -> (w752:bool)  [unwired: 1 in, 1 out]
                n337 = local read "Initialize"() -> (w751:bool)
                n338 = local read "Retract"() -> (w744:bool)
                n339 = local read "Go to Assign Pt"() -> (w748:bool)
                n340 = Compound Arithmetic op=OR(w752, w751, w744) -> (w749:bool)
                n341 = Build Array(w749, w748) -> (w750:bool[])
                n342 = Boolean Array To Number(Boolean array=w750) -> (number=w747:u32)
                n343 = case shown="2" w747 {
                  tunnel: w745 -> [w753 _ _]
                  tunnel: [w753 w754 w757] -> w746
                  frame 0, Default {
                  }
                  frame 1 {
                    w754 = T7."Engaging" ("Current State")
                    n344 = global write "Global Variables.vi" "state changing"(TRUE ("state changing")) -> ()
                    n345 = local write "Initialize"(FALSE ("Initialize")) -> ()
                    n346 = local write "Current System State"(w754) -> ()
                  }
                  frame 2 {
                    w757 = T7."Rerouting" ("Current State")
                    n347 = global write "Global Variables.vi" "state changing"(TRUE ("state changing")) -> ()
                    n348 = local write "Go to Assign Pt"(FALSE ("Initialize")) -> ()
                    n349 = local write "Current System State"(w757) -> ()
                  }
                }
              }
              frame True {
                n350 = local read "To Regulation"() -> (w761:bool)
                n351 = case shown="False" w761 {
                  tunnel: [T7."Tracking" ("Current State") T7."Regulation" ("Current State")] -> w760
                  frame False {
                    n352 = global write "Global Variables.vi" "state changing"(TRUE ("state changing")) -> ()
                  }
                  frame True {
                    n353 = global write "Global Variables.vi" "state changing"(TRUE ("state changing")) -> ()
                  }
                }
                n354 = local write "Current System State"(w760) -> ()
              }
            }
            n355 = global write "Global Variables.vi" "irrigate"(TRUE ("irrigate")) -> ()
          }
          frame "Regulation" {
            n356 = global read "Global Variables.vi" "state flag array"() -> (w770:bool[])
            n357 = global write "Global Variables.vi" "irrigate"(TRUE ("irrigate")) -> ()
            n358 = Index Array(array=w770, index=8) -> (element=w769:bool)
            n359 = case shown="True" w769 {
              tunnel: [w779 w791] -> w768
              tunnel: w767 -> [w778 w792]
              frame False {
                n360 = local read "Initialize"() -> (w777:bool)
                n361 = local read "Retract"() -> (w776:bool)
                n362 = local read "Go to Assign Pt"() -> (w772:bool)
                n363 = Or(x=w777, y=w776) -> (x .or. y?=w775:bool)
                n364 = Build Array(w775, w772) -> (w774:bool[])
                n365 = Boolean Array To Number(Boolean array=w774) -> (number=w773:u32)
                n366 = case shown="2" w773 {
                  tunnel: w778 -> [w780 _ _]
                  tunnel: [w780 w782 w785] -> w779
                  frame 0, Default {
                  }
                  frame 1 {
                    w781 = FALSE  # Reset
                    w782 = T7."Engaging" ("Current State")
                    n367 = global write "Global Variables.vi" "state changing"(TRUE ("state changing")) -> ()
                    n368 = local write "Initialize"(FALSE ("Load Traj")) -> ()
                    n369 = local write "Current System State"(w782) -> ()
                    n370 = local write "To Regulation"(w781) -> ()
                  }
                  frame 2 {
                    w785 = T7."Rerouting" ("Current State")
                    n371 = global write "Global Variables.vi" "state changing"(TRUE ("state changing")) -> ()
                    n372 = local write "Go to Assign Pt"(FALSE ("Initialize")) -> ()
                    n373 = local write "Current System State"(w785) -> ()
                  }
                }
              }
              frame True {
                n374 = local read "Load Traj"() -> (w794:bool)
                n375 = local read "Go to Assign Pt"() -> (w795:bool)
                n376 = local read "Initialize"() -> (w790:bool)
                n377 = local read "Retract"() -> (w788:bool)
                n378 = local read "Track"() -> (w789:bool)
                n379 = Build Array(w794, w795, w790, w788, w789) -> (w796:bool[])
                n380 = Boolean Array To Number(Boolean array=w796) -> (number=w793:u32)
                n381 = case shown="8" w793 {
                  tunnel: w792 -> [w797 _ _ _ _ _]
                  tunnel: [w797 w799 w802 w806 w810 w814] -> w791
                  frame 0, Default {
                  }
                  frame 1 {
                    w798 = FALSE  # Reset
                    w799 = T7."Trajectory Loading" ("Current State")
                    n382 = global write "Global Variables.vi" "state changing"(TRUE ("state changing")) -> ()
                    n383 = local write "Load Traj"(FALSE ("Load Traj")) -> ()
                    n384 = local write "Current System State"(w799) -> ()
                    n385 = local write "To Regulation"(w798) -> ()
                  }
                  frame 2 {
                    w802 = T7."Rerouting" ("Current State")
                    n386 = global write "Global Variables.vi" "state changing"(TRUE ("state changing")) -> ()
                    n387 = local write "Go to Assign Pt"(FALSE ("Load Traj")) -> ()
                    n388 = local write "Current System State"(w802) -> ()
                  }
                  frame 4 {
                    w805 = FALSE  # Reset
                    w806 = T7."Engaging" ("Current State")
                    n389 = global write "Global Variables.vi" "state changing"(TRUE ("state changing")) -> ()
                    n390 = local write "Initialize"(FALSE ("Load Traj")) -> ()
                    n391 = local write "To Regulation"(w805) -> ()
                    n392 = local write "Current System State"(w806) -> ()
                  }
                  frame 8 {
                    w809 = FALSE  # Reset
                    w810 = T7."Aiming" ("Current State")
                    n393 = global write "Global Variables.vi" "state changing"(TRUE ("state changing")) -> ()
                    n394 = local write "Retract"(FALSE ("Load Traj")) -> ()
                    n395 = local write "To Regulation"(w809) -> ()
                    n396 = local write "Current System State"(w810) -> ()
                  }
                  frame 16 {
                    w813 = FALSE  # Reset
                    w814 = T7."Tracking" ("Current State")
                    n397 = global write "Global Variables.vi" "state changing"(TRUE ("state changing")) -> ()
                    n398 = local write "Track"(FALSE ("Load Traj")) -> ()
                    n399 = local write "Current System State"(w814) -> ()
                    n400 = local write "To Regulation"(w813) -> ()
                  }
                }
              }
            }
          }
        }
        n401 = global write "Global Variables.vi" "increment ctrl"("Inc Ctrl") -> ()
        n402 = global write "Global Variables.vi" "z rot axis"("Z Rot Axis") -> ()
        n403 = global write "Global Variables.vi" "reroute transit vacf"("Reroute Transit Vacf") -> ()
        n404 = global write "Global Variables.vi" "vac extremum"("Vac Extremum") -> ()
        n405 = global write "Global Variables.vi" "z dist thld"("Z Dist Thld") -> ()
        n406 = global write "Global Variables.vi" "joint limits"("Joint Limits") -> ()
        n407 = global write "Global Variables.vi" "refractive index"("Refractive Index") -> ()
        n408 = global write "Global Variables.vi" "min AC gap"("Min AC Gap") -> ()
        n409 = global write "Global Variables.vi" "min PC gap"("Min PC Gap") -> ()
        n410 = global write "Global Variables.vi" "reroute hold [sec]"("Reroute Hold [sec]") -> ()
        n411 = global write "Global Variables.vi" "OCT Z cmd Posit"("OCT Cmd Z [mm]") -> ()
        n412 = local read "DH Params"() -> (w380:cluster{"d_DH":dbl[][], "ty":dbl[][]})
        n413 = global read "Global Variables.vi" "irrigate"() -> (w388:bool)
        n414 = call "RisingEdge.vi"("Signal In"="Go to Assign Pt") -> ("Rising Edge"=w402:bool)  [unwired: 10 in]
        n415 = global write "Global Variables.vi" "reset joystick"("Reset Joystick") -> ()
        n416 = global write "Global Variables.vi" "L3 go home"("L3 Go Home") -> ()
        n417 = global write "Global Variables.vi" "stop accurus"("Stop Accurus") -> ()
        n418 = global write "Global Variables.vi" "go to regulation"("To Regulation") -> ()
        n419 = global write "Global Variables.vi" "remote ctrl source"("Remote Control Source") -> ()
        n420 = local write "Go to Assign Pt"(w402) -> ()
        n421 = shared-variable "PXI-Robot\\JointAngles.lvlib\\Eye No"("Eye No") -> ()  [unwired: 1 in, 1 out]
        n422 = global write "var_OCTzHomeDir.vi" "OCTz Home Dir"("OCTz Home Dir") -> ()
        n423 = shared-variable "PXI-Robot\\JointAngles.lvlib\\Irrigation"(w388) -> ()  [unwired: 1 in, 1 out]
        n424 = global write "Global Variables.vi" "Tracking Mode"("Tracking Mode") -> ()
        n425 = global write "Global Variables.vi" "DH Params"(w380) -> ()
        n426 = global read "Global Variables.vi" "armID"() -> (w394:i32)
        n427 = call "RobotDLLError(SubVI).vi"("ArmID"=w394) -> ("RobotStatusArray"=w393:bool[])  [unwired: 5 in, 9 out]
        n428 = global write "Global Variables.vi" "Robot Status Array"(w393) -> ()
        n429 = Index Array(array=w393, index=6) -> (element=w391:bool)
        n430 = Not(x=w391) -> (.not. x?=w390:bool)
        n431 = Number To Decimal String(number="Data No", width (-)=i16 1) -> (decimal integer string=w383:string)
        n432 = shared-variable "PXI-Robot\\JointAngles.lvlib\\Inside RCM"(w390) -> ()  [unwired: 1 in, 1 out]
        n433 = global write "Global Variables.vi" "Inside RCM"(w390) -> ()
        n434 = shared-variable "PXI-Robot\\JointAngles.lvlib\\Data No"(w383) -> ()  [unwired: 1 in, 1 out]
        n435 = shared-variable "PXI-Robot\\JointAngles.lvlib\\Save Data"("Save Data") -> ()  [unwired: 1 in, 1 out]
        n436 = global write "Global Variables.vi" "program stop"("Program Stop") -> ()
      }
      n437 = while {
        tunnel: w72 -> [w160]
        tunnel: w75 -> [w159]
        tunnel: [w158] -> w68
        tunnel: [w157] -> w67
        shift-right: [w155] -> _
        shift-left: 0.0 ("Prev OCT Z Posit") -> [w156]
        shift-right: [w153] -> _
        shift-left: 0 -> [w152]
        shift-right: [w151] -> _
        shift-left: T1 {"Traj Px Array"=[], "Traj Py Array"=[], "Traj Pz Array"=[], "Speed Array"=[], "Depth Array"=[], "Traj Joint1 Array"=[], "Traj Joint2 Array"=[], "Traj Joint3 Array"=[], "Traj Joint4 Array"=[], "Traj Joint5 Array"=[]} ("Trajectory Cluster 2") -> [w149]
        shift-right: [w150] -> _
        shift-left: T4 {"X Grid"=[], "Y Grid"=[], "Za_true Surf"=[], "Iris Center"=[0.0, 5.0, 0.0], "Zp_true Surf"=[], "Pinv"=[[1.0, 0.0], [0.0, 1.0]], "za_true"=0.0, "za_work"=0.0, "zp_work"=0.0, "zp_true"=0.0} ("Eye Model Cluster") -> [w148]
        stop <- w154 stop-if-true
        # "State Execution Loop"
        n438 = Wait (ms)(milliseconds to wait=u32 1) -> ()  [unwired: 1 out]
        n439 = local read "Current System State"() -> (w147:T7)
        n440 = case shown="\"Regulation\"" w147 {
          tunnel: w160 -> [w167 w178 w188 w199 w210 w223 w256 w267 w278 w286]
          tunnel: w159 -> [w163 w174 w183 w194 w205 w220 w252 w261 w272 w281]
          tunnel: [w166 w177 w187 w198 w209 w232 w255 w266 w277 w285] -> w158
          tunnel: [w162 w172 w182 w192 w203 w233 w251 w260 w271 w280] -> w157
          tunnel: w156 -> [_ w176 w185 w196 w207 w221 w253 w263 w274 w283]
          tunnel: [0.0 ("Prev OCT Z Posit") w173 w184 w195 w206 w224 w250 w262 w273 w282] -> w155
          tunnel: [0 ("Last Index") 0 ("Last Index") 0 ("Last Index") 0 ("Last Index") 0 ("Last Index") 0 w249 w264 w275 w289] -> w153
          tunnel: w152 -> [_ _ _ _ _ _ w254 w265 w276 w289]
          tunnel: [T1 {"Traj Px Array"=[], "Traj Py Array"=[], "Traj Pz Array"=[], "Speed Array"=[], "Depth Array"=[], "Traj Joint1 Array"=[], "Traj Joint2 Array"=[], "Traj Joint3 Array"=[], "Traj Joint4 Array"=[], "Traj Joint5 Array"=[]} ("Trajectory Cluster 2") T1 {"Traj Px Array"=[], "Traj Py Array"=[], "Traj Pz Array"=[], "Speed Array"=[], "Depth Array"=[], "Traj Joint1 Array"=[], "Traj Joint2 Array"=[], "Traj Joint3 Array"=[], "Traj Joint4 Array"=[], "Traj Joint5 Array"=[]} ("Trajectory Cluster 2") T1 {"Traj Px Array"=[], "Traj Py Array"=[], "Traj Pz Array"=[], "Speed Array"=[], "Depth Array"=[], "Traj Joint1 Array"=[], "Traj Joint2 Array"=[], "Traj Joint3 Array"=[], "Traj Joint4 Array"=[], "Traj Joint5 Array"=[]} ("Trajectory Cluster 2") T1 {"Traj Px Array"=[], "Traj Py Array"=[], "Traj Pz Array"=[], "Speed Array"=[], "Depth Array"=[], "Traj Joint1 Array"=[], "Traj Joint2 Array"=[], "Traj Joint3 Array"=[], "Traj Joint4 Array"=[], "Traj Joint5 Array"=[]} ("Trajectory Cluster 2") T1 {"Traj Px Array"=[], "Traj Py Array"=[], "Traj Pz Array"=[], "Speed Array"=[], "Depth Array"=[], "Traj Joint1 Array"=[], "Traj Joint2 Array"=[], "Traj Joint3 Array"=[], "Traj Joint4 Array"=[], "Traj Joint5 Array"=[]} ("Trajectory Cluster 2") w231 w248 w257 w268 w288] -> w151
          tunnel: [T4 {"X Grid"=[], "Y Grid"=[], "Za_true Surf"=[], "Iris Center"=[0.0, 5.0, 0.0], "Zp_true Surf"=[], "Pinv"=[[1.0, 0.0], [0.0, 1.0]], "za_true"=0.0, "za_work"=0.0, "zp_work"=0.0, "zp_true"=0.0} ("Eye Model Cluster") T4 {"X Grid"=[], "Y Grid"=[], "Za_true Surf"=[], "Iris Center"=[0.0, 5.0, 0.0], "Zp_true Surf"=[], "Pinv"=[[1.0, 0.0], [0.0, 1.0]], "za_true"=0.0, "za_work"=0.0, "zp_work"=0.0, "zp_true"=0.0} ("Eye Model Cluster") T4 {"X Grid"=[], "Y Grid"=[], "Za_true Surf"=[], "Iris Center"=[0.0, 5.0, 0.0], "Zp_true Surf"=[], "Pinv"=[[1.0, 0.0], [0.0, 1.0]], "za_true"=0.0, "za_work"=0.0, "zp_work"=0.0, "zp_true"=0.0} ("Eye Model Cluster") T4 {"X Grid"=[], "Y Grid"=[], "Za_true Surf"=[], "Iris Center"=[0.0, 5.0, 0.0], "Zp_true Surf"=[], "Pinv"=[[1.0, 0.0], [0.0, 1.0]], "za_true"=0.0, "za_work"=0.0, "zp_work"=0.0, "zp_true"=0.0} ("Eye Model Cluster") T4 {"X Grid"=[], "Y Grid"=[], "Za_true Surf"=[], "Iris Center"=[0.0, 5.0, 0.0], "Zp_true Surf"=[], "Pinv"=[[1.0, 0.0], [0.0, 1.0]], "za_true"=0.0, "za_work"=0.0, "zp_work"=0.0, "zp_true"=0.0} ("Eye Model Cluster") w230 w246 w258 w270 w287] -> w150
          tunnel: w149 -> [_ _ _ _ _ _ w248 w257 w268 w288]
          tunnel: w148 -> [_ _ _ _ _ _ w246 w258 w270 w287]
          frame "Homing", Default {
            n441 = global write "Global Variables.vi" "Tool Offset"("Tool Offset [mm]") -> ()
            n442 = call "Homing Phaco.vi"("error in"=w163, "Tool Offset"="Tool Offset [mm]", "ToolType"="Tool Type", "FPGA VI Reference In"=w167) -> ("error out"=w162:errorcluster, "FPGA VI Reference Out"=w166:refnum<k20>)  [unwired: 6 in]
          }
          frame "M/S Initialization" {
            n443 = local read "OCT Z PID Gains"() -> (w175:cluster{"Kp":dbl, "Kd":dbl, "Ki":dbl})
            n444 = call "MS Initialization Phaco.vi"("OCT Z PID Gains"=w175, "error in"=w174, "OCT Prev Posit"=w176, "FPGA VI Reference In"=w178) -> ("error out"=w172:errorcluster, "OCT Last Posit"=w173:dbl, "FPGA VI Reference Out"=w177:refnum<k20>)  [unwired: 5 in]
          }
          frame "M/S Operation" {
            n445 = local read "OCT Z PID Gains"() -> (w186:cluster{"Kp":dbl, "Kd":dbl, "Ki":dbl})
            n446 = call "MS Operation Phaco.vi"("OCT Z PID Gains"=w186, "error in"=w183, "OCT Prev Posit"=w185, "FPGA VI Reference In"=w188) -> ("error out"=w182:errorcluster, "OCT Last Posit"=w184:dbl, "FPGA VI Reference Out"=w187:refnum<k20>)  [unwired: 5 in]
          }
          frame "Aiming" {
            n447 = local read "OCT Z PID Gains"() -> (w193:cluster{"Kp":dbl, "Kd":dbl, "Ki":dbl})
            n448 = call "Aiming Phaco.vi"("OCT Z PID Gains"=w193, "error in"=w194, "OCT Prev Posit"=w196, "Aiming Pt"="Aiming Pt", "FPGA VI Reference In"=w199) -> ("error out"=w192:errorcluster, "OCT Last Posit"=w195:dbl, "FPGA VI Reference Out"=w198:refnum<k20>)  [unwired: 4 in]
          }
          frame "Engaging" {
            n449 = local read "OCT Z PID Gains"() -> (w204:cluster{"Kp":dbl, "Kd":dbl, "Ki":dbl})
            n450 = call "Engaging Phaco.vi"("OCT Z PID Gains"=w204, "error in"=w205, "OCT Prev Posit"=w207, "Engage Pt"="Engage Pt", "FPGA VI Reference In"=w210) -> ("error out"=w203:errorcluster, "OCT Last Posit"=w206:dbl, "FPGA VI Reference Out"=w209:refnum<k20>)  [unwired: 4 in]
          }
          frame "Trajectory Loading" {
            n451 = local read "OCT Z PID Gains"() -> (w219:cluster{"Kp":dbl, "Kd":dbl, "Ki":dbl})
            n452 = call "Trajectory Loading Phaco.vi"("OCT Z PID Gains"=w219, "error in"=w220, "OCT Prev Posit"=w221, "FPGA VI Reference In"=w223) -> ("error out"=w217:errorcluster, "OCT Last Posit"=w216:dbl, "Trajectory Cluster"=w215:T1, "FPGA VI Reference Out"=w214:refnum<k20>, "Eye Model Cluster"=w218:T4, "First Trk Pt"=→"First Trk Pt":dbl[])  [unwired: 2 in]
            n453 = flat-sequence {
              tunnel: w218 -> [w237]
              tunnel: w217 -> [w239]
              tunnel: [w239] -> w229
              tunnel: w214 -> [w238]
              tunnel: [w238] -> w228
              tunnel: [w235] -> w227
              tunnel: w215 -> [w235]
              tunnel: [w237] -> w226
              tunnel: w216 -> [w236]
              tunnel: [w236] -> w225
              tunnel: [w244] -> w233
              tunnel: w229 -> [w244]
              tunnel: w228 -> [w243]
              tunnel: [w243] -> w232
              tunnel: w227 -> [w242]
              tunnel: w226 -> [w241]
              tunnel: [w242] -> w231
              tunnel: [w241] -> w230
              tunnel: w225 -> [w240]
              tunnel: [w240] -> w224
              frame #0 {
                "Eye Model Cluster" <- w237
                "Trajectory Cluster" <- w235
              }
              frame #1 {
                "Update Mdl & Traj" <- TRUE
              }
            }
          }
          frame "Tracking Initialization" {
            n454 = local read "OCT Z PID Gains"() -> (w247:cluster{"Kp":dbl, "Kd":dbl, "Ki":dbl})
            n455 = call "Tracking Initialization Phaco.vi"("Eye Model Cluster"=w246, "Trajectory Cluster"=w248, "OCT Z PID Gains"=w247, "error in"=w252, "OCT Prev Posit"=w253, "Prev Index"=w254, "FPGA VI Reference In"=w256) -> ("error out"=w251:errorcluster, "OCT Last Posit"=w250:dbl, "Last Index"=w249:i32, "FPGA VI Reference Out"=w255:refnum<k20>)  [unwired: 1 in]
          }
          frame "Tracking" {
            n456 = local read "OCT Z PID Gains"() -> (w259:cluster{"Kp":dbl, "Kd":dbl, "Ki":dbl})
            n457 = call "Tracking Phaco.vi"("Trajectory Cluster"=w257, "OCT Z PID Gains"=w259, "Eye Model Cluster"=w258, "error in"=w261, "OCT Prev Posit"=w263, "Resume Index"=w265, "FPGA VI Reference In"=w267) -> ("error out"=w260:errorcluster, "OCT Last Posit"=w262:dbl, "Leave Index"=w264:i32, "FPGA VI Reference Out"=w266:refnum<k20>)  [unwired: 1 in]
          }
          frame "Rerouting" {
            n458 = local read "OCT Z PID Gains"() -> (w269:cluster{"Kp":dbl, "Kd":dbl, "Ki":dbl})
            n459 = call "Rerouting Phaco.vi"("Eye Model Cluster"=w270, "Trajectory Cluster"=w268, "OCT Z PID Gains"=w269, "error in"=w272, "OCT Prev Posit"=w274, "Prev Index"=w276, "FPGA VI Reference In"=w278) -> ("error out"=w271:errorcluster, "OCT Last Posit"=w273:dbl, "Last Index"=w275:i32, "FPGA VI Reference Out"=w277:refnum<k20>)  [unwired: 1 in]
          }
          frame "Regulation" {
            n460 = local read "OCT Z PID Gains"() -> (w279:cluster{"Kp":dbl, "Kd":dbl, "Ki":dbl})
            n461 = local read "Engage Pt"() -> (w284:dbl[])
            n462 = call "Regulation Phaco.vi"("OCT Z PID Gains"=w279, "error in"=w281, "OCT Prev Posit"=w283, "Engage Pt"=w284, "FPGA VI Reference In"=w286) -> ("error out"=w280:errorcluster, "OCT Last Posit"=w282:dbl, "FPGA VI Reference Out"=w285:refnum<k20>)  [unwired: 4 in]
          }
        }
        n463 = local read "Program Stop"() -> (w154:bool)
      }
      n464 = while {
        tunnel: w77 -> [w322]
        tunnel: [w321] -> w76
        stop <- w331 stop-if-true
        # "Indicator Loop"
        n465 = global read "Global Variables.vi" "armID"() -> (w297:i32)
        n466 = Wait (ms)(milliseconds to wait=u32 100) -> ()  [unwired: 1 out]
        n467 = global read "Global Variables.vi" "L1 to L4 cmd Posit"() -> (w303:dbl[])
        n468 = global read "Global Variables.vi" "L1 to L4 out Posit"() -> (w296:dbl[])
        "Joint Out" <- w296
        n469 = global read "Global Variables.vi" "DH Params"() -> (w290:cluster{"d_DH":dbl[][], "ty":dbl[][]})
        n470 = Index Array(array=w303) -> (element #1=w302:dbl, element #2=w301:dbl, element #3=w300:dbl, element #4=w298:dbl)  [unwired: 4 in]
        n471 = Index Array(array=w296) -> (element #1=w295:dbl, element #2=w294:dbl, element #3=w293:dbl, element #4=w292:dbl)  [unwired: 4 in]
        n472 = call "Forward Kinematics with DH.vi"("DH Params"=w290, "j4"=w298, "j3"=w300, "j2"=w301, "j1"=w302, "armID"=w297) -> ("XYZ With DH Calibration"=→"Tip cmd Posit":dbl[])  [unwired: 5 in]
        n473 = call "Forward Kinematics with DH.vi"("DH Params"=w290, "j4"=w292, "j3"=w293, "j2"=w294, "j1"=w295, "armID"=w297) -> ("XYZ With DH Calibration"=w291:dbl[])  [unwired: 5 in]
        "Tip out Posit" <- w291
        n474 = shared-variable "PXI-Robot\\JointAngles.lvlib\\ToolTipPosition"(w291) -> ()  [unwired: 1 in, 1 out]
        n475 = global write "Global Variables.vi" "Tip out Posit"(w291) -> ()
        n476 = global read "Global Variables.vi" "Stage cmd Posit"() -> (→"XYZ Stage cmd":dbl[])
        n477 = global read "Global Variables.vi" "Stage out Posit"() -> (w306:dbl[])
        "XYZ Stage out" <- w306
        n478 = global read "Global Variables.vi" "OCT Z out Posit"() -> (→"OCT Z out [mm]":dbl)
        n479 = global read "Global Variables.vi" "L5 out Posit"() -> (→"Grasp out":dbl)
        n480 = Index Array(array=w306) -> (element #3=w307:dbl)  [unwired: 3 in, 2 out]
        n481 = shared-variable "PXI-Robot\\JointAngles.lvlib\\Stage Z Out"(w307) -> ()  [unwired: 1 in, 1 out]
        n482 = global read "Global Variables.vi" "irrigate"() -> (→"Irrigation Engaged?":bool)
        n483 = global read "Global Variables.vi" "vac digit cmd"() -> (w312:i8)
        n484 = global read "Global Variables.vi" "max limit [mmHg]"() -> (w309:dbl)
        n485 = global read "Global Variables.vi" "Robot Status Array"() -> (→"Robot Status Array":bool[])
        n486 = global read "Global Variables.vi" "Robot Home Status"() -> (→"Status 2":bool[])
        n487 = global read "Global Variables.vi" "Receive Count"() -> (→"Receive Count":u64)
        n488 = global read "Global Variables.vi" "Send Count"() -> (→"Send Count":u64)
        n489 = global read "Global Variables.vi" "current run no."() -> (→"Current Run No.":u8)
        n490 = Divide(x=w312, y=i8 78) -> (x/y=w310:dbl)
        n491 = Multiply(x=w310, y=w309) -> (x*y=→"Value [mmHg]" →"Vacuum Force [mmHg]  2":dbl)
        n492 = shared-variable "PXI-Robot\\JointAngles.lvlib\\RemoteSenderEngaged"() -> (→"Remote sender engaged":bool)  [unwired: 1 in, 1 out]
        n493 = shared-variable "PXI-Robot\\JointAngles.lvlib\\EmergencyAlarmBit"() -> (→"Emergency alarm":bool)  [unwired: 1 in, 1 out]
        n494 = global read "Global Variables.vi" "assign pt out of bound"() -> (→"Asgn Pt Out of Bound":bool)
        n495 = global read "Global Variables.vi" "tracking timer"() -> (w324:i32)
        n496 = global read "Global Variables.vi" "state changing"() -> (→"State changing":bool)
        n497 = global read "Global Variables.vi" "state flag array"() -> (→"State Flag Array":bool[])
        n498 = Divide(x=w324, y=10) -> (x/y=→"Timer":dbl)
        n499 = flat-sequence {
          frame #0 {
            w353 = sgl[] [0.0, 0.0]  # RCMy
            w352 = sgl[] [0.0, 0.0]  # RCMz
            w354 = sgl[] [0.0, 0.0]  # RCMx
            # "3D Visualization"
            n500 = disable-structure shown="Disabled" {
              disable-tunnel: [w363 _] -> w342
              frame Disabled {
                n501 = global read "Global Variables.vi" "xPC"() -> (w361:dbl[])
                n502 = global read "Global Variables.vi" "yPC"() -> (w360:dbl[])
                n503 = global read "Global Variables.vi" "zPC"() -> (w359:dbl[])
                n504 = call-poly <vilib>:"Plot Helper.vi"("Plot ID"=2, "z vector"=w359, "y vector"=w360, "x vector"=w361) -> ("3D Plot lvclass Array out"=w368:refnum<class "3D Plot Datatype.lvclass">[])  [unwired: 2 in, 5 out]
                n505 = global read "Global Variables.vi" "xACh"() -> (w366:dbl[])
                n506 = global read "Global Variables.vi" "yACh"() -> (w365:dbl[])
                n507 = global read "Global Variables.vi" "zACh"() -> (w364:dbl[])
                n508 = call-poly <vilib>:"Plot Helper.vi"("Plot ID"=3, "z vector"=w364, "y vector"=w365, "x vector"=w366, "3D Plot lvclass Array in"=w368) -> ("3D Plot lvclass Array out"=w363:refnum<class "3D Plot Datatype.lvclass">[])  [unwired: 1 in, 5 out]
              }
              frame Enabled {
              }
            }
            n509 = local read "Tip out Posit"() -> (w346:dbl[])
            n510 = call "Vis Interpolate Points.vi"("Tip out Posit"=w346) -> ("Z"=w343:dbl[], "Y"=w344:dbl[], "X"=w345:dbl[])  [unwired: 4 in]
            n511 = call-poly <vilib>:"Plot Helper.vi"("Plot ID"=1, "z vector"=w343, "y vector"=w344, "x vector"=w345, "3D Plot lvclass Array in"=w342) -> ("3D Plot lvclass Array out"=w336:refnum<class "3D Plot Datatype.lvclass">[])  [unwired: 1 in, 5 out]
            n512 = global read "Global Variables.vi" "xTraj"() -> (w337:dbl[])
            n513 = global read "Global Variables.vi" "yTraj"() -> (w338:dbl[])
            n514 = global read "Global Variables.vi" "zTraj"() -> (w339:dbl[])
            n515 = call-poly <vilib>:"Plot Helper.vi"("Plot ID"=4, "z vector"=w339, "y vector"=w338, "x vector"=w337, "3D Plot lvclass Array in"=w336) -> ("3D Plot lvclass Array out"=w334:refnum<class "3D Plot Datatype.lvclass">[])  [unwired: 1 in, 5 out]
            n516 = disable-structure shown="Disabled" {
              disable-tunnel: w334 -> [w370 w375]
              disable-tunnel: [w369 w375] -> w333
              frame Disabled {
                n517 = global read "Global Variables.vi" "xIris"() -> (w374:dbl[])
                n518 = global read "Global Variables.vi" "yIris"() -> (w373:dbl[])
                n519 = global read "Global Variables.vi" "zIris"() -> (w372:dbl[])
                n520 = call-poly <vilib>:"Plot Helper.vi"("Plot ID"=6, "z vector"=w372, "y vector"=w373, "x vector"=w374, "3D Plot lvclass Array in"=w370) -> ("3D Plot lvclass Array out"=w369:refnum<class "3D Plot Datatype.lvclass">[])  [unwired: 1 in, 5 out]
              }
              frame Enabled {
              }
            }
            n521 = Index Array(array=w346) -> (element #1=w357:dbl, element #2=w356:dbl, element #3=w355:dbl)  [unwired: 3 in]
            n522 = Build Array (concatenate)(w354, w357) -> (w349:dbl[])
            n523 = Build Array (concatenate)(w353, w356) -> (w348:dbl[])
            n524 = Build Array (concatenate)(w352, w355) -> (w347:dbl[])
            n525 = call-poly <vilib>:"Plot Helper.vi"("Plot ID"=5, "z vector"=w347, "y vector"=w348, "x vector"=w349, "3D Plot lvclass Array in"=w333) -> ("3D Plot lvclass Array out"=w340:refnum<class "3D Plot Datatype.lvclass">[])  [unwired: 1 in, 5 out]
            n526 = call-poly <vilib>:"Plot Helper.vi"("Plot ID"=6, "z vector"=w352, "y vector"=w353, "x vector"=w354, "3D Plot lvclass Array in"=w340) -> ("3D Plot lvclass Array out"=→"Robot XYZ":refnum<class "3D Plot Datatype.lvclass">[])  [unwired: 1 in, 5 out]
          }
        }
        n527 = local read "Current System State"() -> (w320:T7)
        n528 = disable-structure shown="Disabled" {
          disable-tunnel: w322 -> [w379 _]
          disable-tunnel: [w378 _] -> w321
          disable-tunnel: w320 -> [w377 _]
          frame Disabled {
            # "Disable write to mitigate finished late"
            n529 = local read "Online Eye Model"() -> (w376:T2)
            n530 = call "WriteLog.vi"("Online Eye Model"=w376, "Current System State"=w377, "File In"=w379) -> ("File Out"=w378:refnum<file>)  [unwired: 8 in]
          }
          frame Enabled {
          }
        }
        n531 = local read "Program Stop"() -> (w331:bool)
        n532 = shared-variable "PXI-Robot\\JointAngles.lvlib\\SystemState"(w320) -> ()  [unwired: 1 in, 1 out]
      }
      n533 = while {
        shift-right: [w96] -> _
        shift-left: errorcluster {"status"=FALSE, "code"=0, "source"=""} ("error IO") -> [w101]
        stop <- w99 stop-if-true
        # "Eye Model and Trajectory Generation"
        n534 = Wait (ms)(milliseconds to wait=u32 100) -> ()  [unwired: 1 out]
        n535 = event shown="[3] \"Gen Traj\": Mouse Up" {
          selector: _ -> [_ _ _ _]
          dyn-events: _ -> [_ _ _ _]
          timeout: 100 -> [_ _ _ _]
          tunnel: [w107 w108 errorcluster {"status"=FALSE, "code"=0, "source"=""} ("error IO") w139] -> w96
          tunnel: w101 -> [w107 w111 _ w139]
          tunnel: "SCAN_NO" -> [_ w112 _ w138]
          event Timeout {
            # "timeout"
            n536 = event-data() -> ()  [unwired: 1 in, 1 out]
          }
          event "Process VSCAN": Value Change {
            # "run ML script to segment the vscan (ACh or PC)"
            n537 = event-data() -> ()  [unwired: 1 in, 2 out]
            n538 = flat-sequence {
              tunnel: w112 -> [w116]
              tunnel: w111 -> [w115]
              tunnel: [w114] -> w110
              tunnel: w110 -> [w120]
              tunnel: [w120] -> w109
              tunnel: w109 -> [w123]
              tunnel: [w122] -> w108
              frame #0 {
                n539 = disable-structure shown="Disabled" {
                  disable-tunnel: w116 -> [w119 _]
                  disable-tunnel: w115 -> [w118 _]
                  disable-tunnel: [w117 _] -> w114
                  frame Disabled {
                    n540 = script code="% 2021-09-20 MJG \n% Segment vscan, generate {OCT} [mm] plot, and save all model parameters\ncd('D:\\IRISSoft LV2016 beta\\Host Demo\\Traj\\BuildModel\\matlab');\n\nclear processVSCAN_v3;\nprocessVSCAN_v3(SCAN_NO_ACh);"("??"=w118, "SCAN_NO_ACh"=w119) -> ("??"=w117:errorcluster)
                  }
                  frame Enabled {
                  }
                }
              }
              frame #1 {
                n541 = disable-structure shown="Disabled" {
                  frame Disabled {
                    w121 = dbl[] [0.0, 0.0, 0.0, 0.0] ("First Trk Pt 2")
                    n542 = global write "Global Variables.vi" "xPC"(w121) -> ()
                    n543 = global write "Global Variables.vi" "yPC"(w121) -> ()
                    n544 = global write "Global Variables.vi" "zPC"(w121) -> ()
                    n545 = global write "Global Variables.vi" "xACh"(w121) -> ()
                    n546 = global write "Global Variables.vi" "yACh"(w121) -> ()
                    n547 = global write "Global Variables.vi" "zACh"(w121) -> ()
                  }
                  frame Enabled {
                  }
                }
              }
              frame #2 {
                n548 = disable-structure shown="Disabled" {
                  disable-tunnel: w123 -> [w128 _]
                  disable-tunnel: [w127 _] -> w122
                  frame Disabled {
                    n549 = local read "SCAN_NO"() -> (w132:string)
                    n550 = script code="cd('D:\\IRISSoft LV2016 beta\\Host Demo\\Traj');\nclear visMdlInLV;\n[xACh, yACh, zACh, xIris, yIris, zIris, xPC, yPC, zPC] = visMdlInLV(SCAN_NO);"("??"=w128, "SCAN_NO"=w132) -> ("??"=w127:errorcluster, "xACh"=w133:dbl[], "yACh"=w134:dbl[], "zACh"=w135:dbl[], "xPC"=w131:dbl[], "yPC"=w130:dbl[], "zPC"=w129:dbl[], "xIris"=w126:dbl[], "yIris"=w125:dbl[], "zIris"=w124:dbl[])
                    n551 = global write "Global Variables.vi" "xACh"(w133) -> ()
                    n552 = global write "Global Variables.vi" "yACh"(w134) -> ()
                    n553 = global write "Global Variables.vi" "zACh"(w135) -> ()
                    n554 = global write "Global Variables.vi" "xIris"(w126) -> ()
                    n555 = global write "Global Variables.vi" "yIris"(w125) -> ()
                    n556 = global write "Global Variables.vi" "zIris"(w124) -> ()
                    n557 = global write "Global Variables.vi" "xPC"(w131) -> ()
                    n558 = global write "Global Variables.vi" "yPC"(w130) -> ()
                    n559 = global write "Global Variables.vi" "zPC"(w129) -> ()
                  }
                  frame Enabled {
                  }
                }
              }
            }
            n560 = disable-structure shown="Disabled" {
              frame Disabled {
                "Model Created" <- TRUE ("Model Created")
              }
              frame Enabled {
              }
            }
          }
          event "Restart": Mouse Up {
            n561 = event-data() -> ()  [unwired: 1 in, 2 out]
          }
          event "Gen Traj": Mouse Up {
            # "Generate trajectory"
            n562 = event-data() -> ()  [unwired: 1 in, 2 out]
            n563 = disable-structure shown="Disabled" {
              disable-tunnel: w138 -> [w146 _]
              disable-tunnel: "Current Surgical Stage" -> [w140 _]
              frame Disabled {
                n564 = call "Update Trajectory.vi"("Current Surgical Stage"=w140, "Pattern"="Pattern", "Depth Ctrl Array\n(% Thickness)"="Depth Ctrl Array\n(% Thickness)", "Scale"="Radial Scale", "Offset"="Offset", "SCAN_NO"=w146) -> ("Trajectory OOB"=→"Trajectory OOB":bool)  [unwired: 5 in]
              }
              frame Enabled {
              }
            }
          }
        }
        "Generation Error" <- w96
        n565 = case shown="True" "Use Online Scan" {
          frame False {
            # "User specified SCAN_NO"
          }
          frame True {
            # "Use the SCAN_NO from OCT computer"
            n566 = shared-variable "PXI-Robot\\JointAngles.lvlib\\SCAN_NO"() -> (w106:string)  [unwired: 1 in, 1 out]
            n567 = local write "SCAN_NO"(w106) -> ()
          }
        }
        n568 = shared-variable "PXI-Robot\\JointAngles.lvlib\\Scan Done"() -> (w97:bool)  [unwired: 1 in, 1 out]
        n569 = case shown="True" w97 {
          frame False {
          }
          frame True {
            n570 = property on="Process VSCAN" class="Bool (strict)"() -> ("Value"=w105:bool)  [unwired: 2 in, 2 out]
            n571 = Not(x=w105) -> (.not. x?=w104:bool)
            n572 = property on="Process VSCAN" class="Bool (strict)"("Val(Sgnl)"=w104) -> ()  [unwired: 2 in, 2 out]
            n573 = shared-variable "PXI-Robot\\JointAngles.lvlib\\Scan Done"(FALSE ("Scan Done")) -> ()  [unwired: 1 in, 1 out]
          }
        }
        n574 = local read "Program Stop"() -> (w99:bool)
      }
      n575 = while {
        tunnel: w63 -> [w92]
        stop <- w93 stop-if-true
        # "Robot Communication Loop (100 Hz)"
        n576 = Wait (ms)(milliseconds to wait=u32 1) -> ()  [unwired: 1 out]
        n577 = global read "Global Variables.vi" "L1 to L4 cmd Posit"() -> (w79:dbl[])
        n578 = global read "Global Variables.vi" "Stage cmd Posit"() -> (w88:dbl[])
        n579 = global read "Global Variables.vi" "L5 M/S cmd"() -> (w81:dbl)
        n580 = shared-variable "PXI-Robot\\JointAngles.lvlib\\L1 to L4 Cmd"(w79) -> ()  [unwired: 1 in, 1 out]
        n581 = call "MS IRISS V2.vi"("Stage Cmd Posit"=w88, "L5 cmd Posit"=w81, "Joint Cmd Posit"=w79, "ArmID"=w92) -> ("Stage Out Posit"=w87:dbl[], "L5 Out Posit"=w82:dbl, "Joint Out Posit"=w80:dbl[], "Connection Status"=→"Status":bool, "Receive Count"=w89:u64, "Send Count"=w90:u64)  [unwired: 2 in]
        n582 = global write "Global Variables.vi" "L1 to L4 out Posit"(w80) -> ()
        n583 = global write "Global Variables.vi" "L5 out Posit"(w82) -> ()
        n584 = global write "Global Variables.vi" "Stage out Posit"(w87) -> ()
        n585 = global write "Global Variables.vi" "Receive Count"(w89) -> ()
        n586 = global write "Global Variables.vi" "Send Count"(w90) -> ()
        n587 = shared-variable "PXI-Robot\\JointAngles.lvlib\\L1 to L4 Out"(w80) -> ()  [unwired: 1 in, 1 out]
        n588 = Index Array(array=w80, index=2) -> (element=w85:dbl)
        n589 = Greater?(x=w85, y=0.05) -> (0:w84:bool)
        n590 = global write "Global Variables.vi" "irrigate"(w84) -> ()
        n591 = local read "Program Stop"() -> (w93:bool)
      }
      n592 = Build Array(w64, w64, w64, w64, w64, w64, w64, w64) -> (w65:i16[])
      n593 = xnode "Output Shut Down"("FPGA VI Reference In"=w68, "error in"=w67, "AO"=w65, "INHB X"=w66, "INHB Y"=w66, "INHB Z"=w66, "INHB OCT Mot"=w66) -> ("FPGA VI Reference Out"=w74:refnum<k20>, "error out"=w73:errorcluster)
    }
    frame #3 {
      # "Reset Flags"
      n594 = disable-structure shown="Disabled" {
        disable-tunnel: w820 -> [w821 _]
        frame Disabled {
          n595 = Close File(refnum=w821) -> ()  [unwired: 1 in, 2 out]
        }
        frame Enabled {
        }
      }
      n596 = global write "Global Variables.vi" "irrigate"(FALSE ("irrigate")) -> ()
    }
    frame #4 {
      # "Close Application"
      n597 = xnode "FPGA Reset"("FPGA VI Reference In"=w827, "error in"=w826) -> ("FPGA VI Reference Out"=w822:refnum<k20>, "error out"=w823:errorcluster)
      n598 = global read "Global Variables.vi" "armID"() -> (w825:i32)
      n599 = dll-call lib="D:/Kevin/IRISS V2 dev/Host Demo/Functions/EyeRobotDLL.dll" fn="CloseRobot" label="Close"("id"=w825) -> ()  [unwired: 5 in, 2 out]
      n600 = xnode "Close FPGA VI Reference"("FPGA VI Reference In"=w822, "error in"=w823) -> ("error out"=→"Error(s) Out on Program End":errorcluster)
    }
  }
